vi "Main_Andor_Multi_ver1.vi"() -> ()   [LabVIEW 2014]
doc: "This is the main user interface of the Raman spectroscopy system."
uses:
  C:/Users/light/Desktop/Chuanzhen/Labview/Raman/dll/Thorlabs.MotionControl.Controls.dll
  dll/Thorlabs.MotionControl.Controls.dll
  <userlib>/atmcd64d.llb/AcquisitionMode_mode typedef.ctl
  <userlib>/atmcd64d.llb/ReadMode_mode typedef.ctl
  <userlib>/atmcd64d.llb/Shutter_mode typedef.ctl
  <userlib>/atmcd64d.llb/Shutter_type typedef.ctl
  <userlib>/atmcd64d.llb/TriggerMode_mode typedef.ctl
  TypeDef/GalvoInput.ctl
  <userlib>/atmcd64d.llb/Error Code Enum typedef.ctl
  TypeDef/States.ctl
  TypeDef/StageDeviceOut.ctl
  TypeDef/StageHandleIn.ctl
  <vilib>/Utility/miscctls.llb/LVPoint32TypeDef.ctl
  TypeDef/LaserSpot.ctl
  C:/Users/light/Desktop/Chuanzhen/Labview/Raman/dll/ThorLabs.MotionControl.KCube.DCServoCLI.dll
  dll/ThorLabs.MotionControl.KCube.DCServoCLI.dll
  TypeDef/StageSelect.ctl
  TypeDef/inputImages.ctl
  C:/Users/light/Desktop/Chuanzhen/Labview/Raman/dll/Thorlabs.MotionControl.GenericMotorCLI.dll
  dll/Thorlabs.MotionControl.GenericMotorCLI.dll
panel:
  out "Boolean":bool
  in  "Tab Control":enum32{"Main", "Andor", "Galvo"}(tab)
  in  "Galvo DC":bool
  out "Galvo":bool
  out "Spot Y":dbl
  out "Spot X":dbl
  in  "Box":cluster{"Width":dbl, " Height":dbl}={"Width"=200.0, " Height"=214.0}
  in  "Quit":bool
  out "Height":i32=480
  out "Width":i32=640
  out "FPS":dbl=6.258409738085552
  in  "Blacklevel Offset":i32(slide) min=0 max=255 scale=0.0..255.0
  in  "Frame rate":dbl(slide)=30.0 min=0.5 max=17.288905497022668 step=5.487719298245614e-05 scale=0.5..17.288905497022668 scale format="%^#_3g"
  in  "Pixel clock":i32(slide)=20 min=7 max=86 scale=7.0..86.0
  in  "Exposure time (ms)":dbl(slide)=11.094175438596492 min=0.008982456140350877 max=107.28491228070176 step=0.05487719298245614 scale=0.008982456140350877..107.28491228070176 scale format="%#.3g"
  in  "Edge Filter Enable / Disable":bool
  in  "Edge Filter":i32(ring)=2 items=["High"=1, "Low"=2]
  in  "Blacklevel compensation":bool
  in  "Hotpixel correction 2":bool
  in  "Master Gain":i32(slide) min=0 max=100 scale=0.0..100.0
  in  "Autogain":bool
  out "Bits/Pixel":i32=8
  in  "Camera ID":u32
  in  "Scan Mode":bool
  out "Live video":picture caption="600 x 480"
  in  "Focus":bool
  out "ZoomRatio":dbl format="%#_2g"
  in  "Jog size (um)":dbl=2.0
  out "Delay (s)":dbl=0.9 format="%#_13g"
  out "Focal plane (mm)":dbl
  out "Initialization finished":bool
  in  "Aim":bool
  in  "Pixel Size X (um)":dbl=0.0877
  in  "LaserSpot":bool
  in  "Pixel Size Y (um)":dbl=0.0877
  in  "Snap":bool
  in  "Left":bool
  in  "Right":bool
  in  "Up":bool
  in  "Down":bool
  in  "X axis_R":bool
  in  "X axis_L":bool
  in  "Reset":bool
  out "Z_axis":dbl
  out "X_axis":dbl
  out "Y_axis":dbl
  in  "Y axis_B":bool
  in  "Y axis_F":bool
  in  "Z axis_u":bool
  in  "Z axis_d":bool
  in  "Jogstep of Z axis":T1(radio)=enum."10step"
  in  "MoveTo":bool
  in  "Velocity: X and Y axis":T2(radio)=enum."0.05mm"
  in  "Scan":bool
  in  "Save Path":path=path "C:/Users/light/Desktop/Chuanzhen/test"
  in  "Destination":dbl=12.0
  out "Frame_X":dbl
  out "Frame_Y":dbl
  out "Total_Frame_X":dbl
  out "Total_Frame_Y":dbl
  in  "Galvo Stop":bool
  in  "Galvo Scan":bool
  out "Andor":bool
  in  "Delay/ms":u32=500
  in  "Set":bool
  in  "AndorSnap":bool
  out "SaveStatus":bool
  in  "FilePath":string="C:\\Users\\light\\Desktop\\Chuanzhen\\Image\\ImageReconstruct\\data"
  in  "Exit":bool
  out "ShutDown":cluster{"CoolOff":bool, "ShutDown":bool}
  in  "Mode":T8={"AcqMode"=enum."Single Scan", "ReadMode"=enum."Single-Track", "ShutterMode"=enum."Auto", "GateMode"=enum."TTL High", "TriggerMode"=enum."Internal"}
  in  "AcqSet":T9={"openingtime"=15, "closingtime/ms"=15, "ExposureTime/s"=0.1, "AccumCycTime"=0.0, "AccumCycNum"=1, "KineticNum"=1, "KineticTime"=0.0} {"KineticTime" format="%.5f"; "AccumCycNum" format="%.5f"; "AccumCycTime" format="%.5f"; "ExposureTime/s" format="%.5f"; "closingtime/ms" format="%.2f"; "openingtime" format="%.2f"}
  out "Timing":T10 {"kinetic" format="%.7f"; "accumulate" format="%.7f"; "exposure" format="%.7f"}
  out "SetOut":T11
  in  "MultiTrack":cluster{"StartRow":i32, "EndRow":i32}={"StartRow"=131, "EndRow"=143}
  out "SetStatus":bool
  out "CurrentTemp":i32
  out "DevInit":bool
  out "DevSize":cluster{"xpixels":i32, "ypixels":i32}
  out "HardWVersion":T12
  out "SoftWVersion":T13
  out "Speeds":T14
  in  "TargetTemp":i32=-70
  out "CoolerON":T15
  out "GetStatus":T16
  in  "YOffset":dbl=8.2 caption="Offset"
  in  "XOffset":dbl=4.0 caption="Offset"
  out "Sample Rate":dbl=1000.0 format="%0.2f"
  out "Waveform Graph":waveform(dbl)[](graph)=[{"t0"=timestamp(0 s since 1904-01-01), "dt"=0.001, "Y"=[]}]
  in  "ZOffset":dbl caption="Offset"
  in  "Galvo":T17={"Sample Rate"=50.0, "Sample Clock Source"="OnboardClock", "Max Voltage"=10.0, "Min Voltage"=-10.0, "Physical Channel(s)"="Dev1/ao0,Dev1/ao1,Dev1/ao3"}
  in  "Stage Control":enum32{"X axis", "Y axis", "Z axis"}(tab)
  in  "X axis":refnum<k24>(container)
  in  "Y axis":refnum<k24>(container)
  in  "Z axis":refnum<k24>(container)
  # "Camera Control"
  # "Objective: CFI Plan Fluor ELWD 60x (1.27 NA) \nThe depth of field: 1.78 um\nPixel Size: 0.0877um/px"
  # "Attention: \ndon't click button very fast"
  # "Motor Control"
  # "Aim"
  # "Auto Focus"
  # "Adjust laser spot lightly"
  # "Stage Scan"
  # "Total_Frame"
  # "Current_Frame"
  # "X"
  # "Y"
  # "Focus distance ia about 2mm"
  # "Jogstep:"
  # "0.00003mm/step"
  # "Stepsize:"
  # "Kinetics->SignleTrack"
  # "Galvo Control"
  # "50Hz->1s"
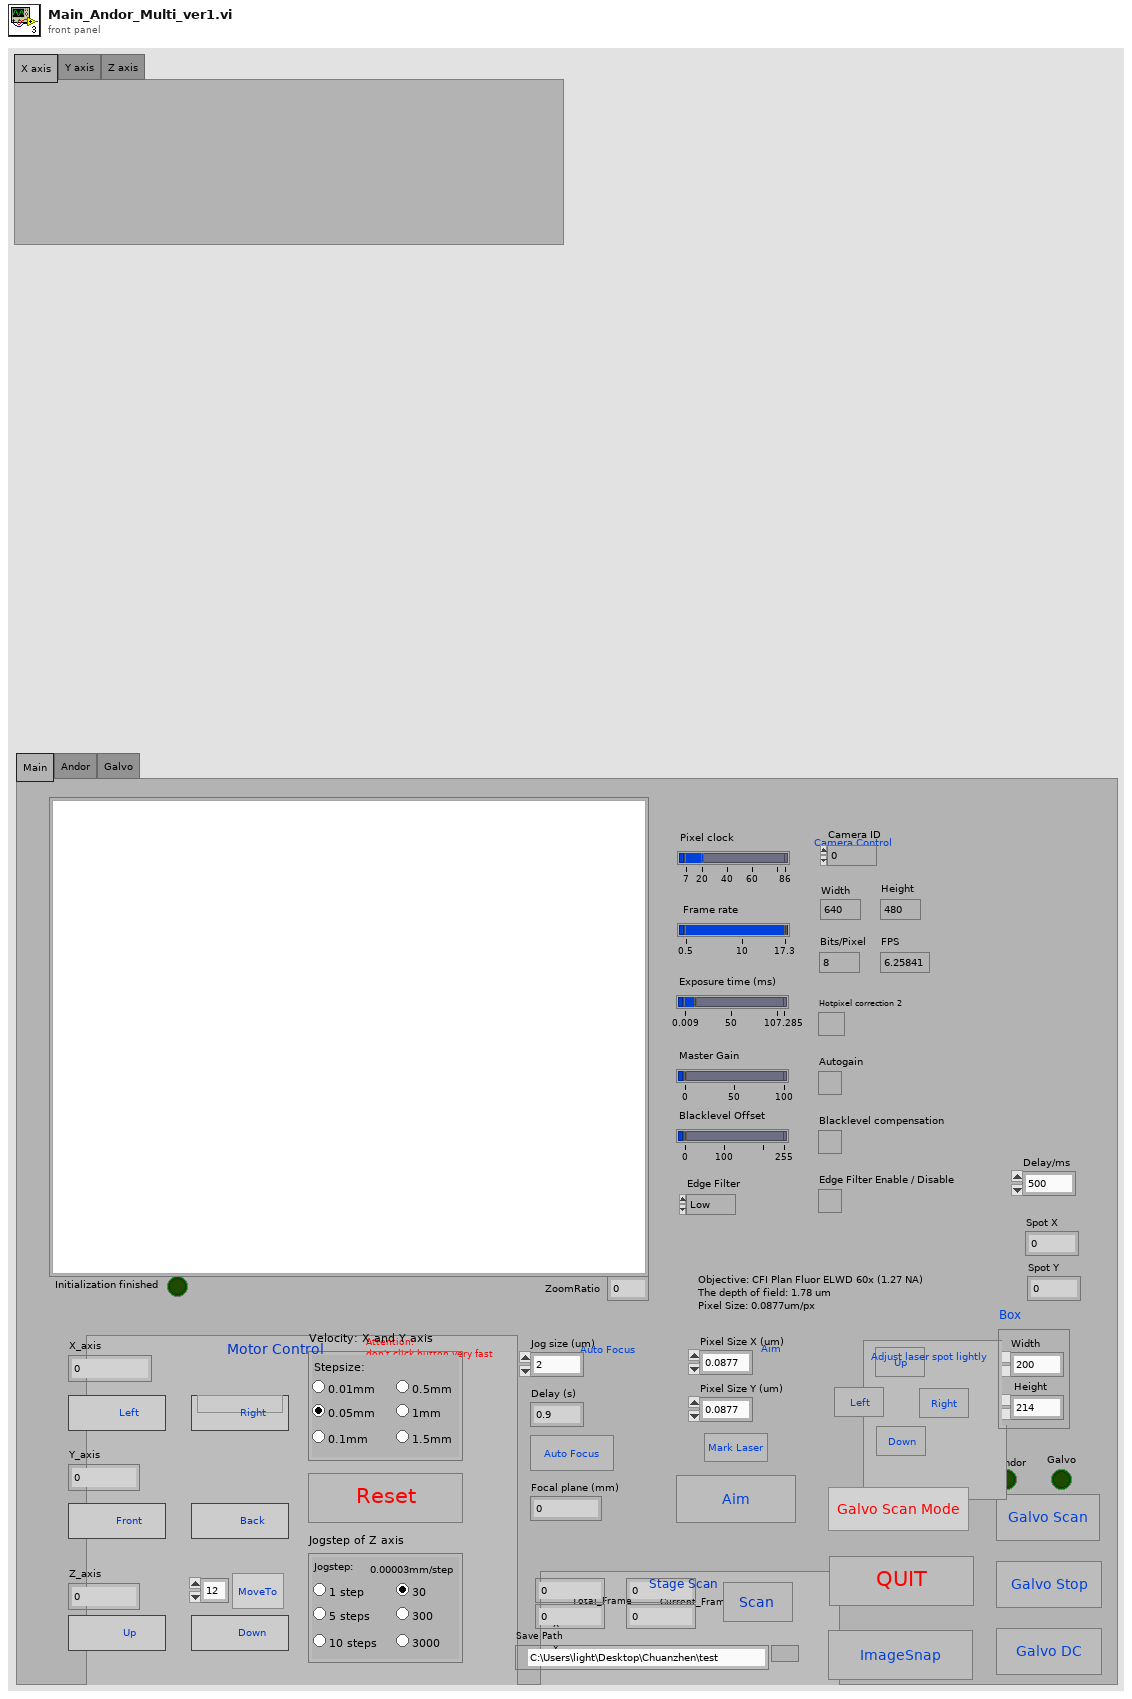
[diagram p1: front panel]
types:
  T1 = enum32{"1step", "2step", "5step", "10step", "15step", "20step"}
  T2 = enum32{"0.01mm", "0.05mm", "0.1mm", "0.5mm", "1mm", "1.5mm"}
  T3 = typedef "AcquisitionMode_mode typedef.ctl" = enum16{"Reserved (0)", "Single Scan", "Accumulate", "Kinetics", "Fast Kinetics", "Run Till Abort", "Reserved (6)", "Reserved (7)", "Reserved (8)", "Time Delayed Integration"}
  T4 = typedef "ReadMode_mode typedef.ctl" = enum16{"Full Vertical Binning", "Multi-Track", "Random-Track", "Single-Track", "Image"}
  T5 = typedef "Shutter_mode typedef.ctl" = enum16{"Auto", "Open", "Close", "N/A (3)", "Open FVB Series", "Open Any Series"}
  T6 = typedef "Shutter_type typedef.ctl" = enum16{"TTL Low", "TTL High"}
  T7 = typedef "TriggerMode_mode typedef.ctl" = enum16{"Internal", "External", "N/A (2)", "N/A (3)", "N/A (4)", "N/A (5)", "External Start", "External Exposure (Bulb)", "N/A (8)", "External FVB EM", "Software", "N/A (11)", "External Charge Shifting"}
  T8 = cluster{"AcqMode":T3, "ReadMode":T4, "ShutterMode":T5, "GateMode":T6, "TriggerMode":T7}
  T9 = cluster{"openingtime":i32, "closingtime/ms":i32, "ExposureTime/s":sgl, "AccumCycTime":sgl, "AccumCycNum":i32, "KineticNum":i32, "KineticTime":sgl}
  T10 = cluster{"exposure":sgl, "accumulate":sgl, "kinetic":sgl}
  T11 = cluster{"Height":i32, "Width":i32, "bottom":i32, "gap":i32}
  T12 = cluster{"PCB":u32, "Flex":u32, "dummy1":u32, "dummy2":u32, "dummy3":u32, "dummy4":u32}
  T13 = cluster{"eprom":u32, "cofFile":u32, "vxdRev":u32, "vxdVer":u32, "dllRev":u32, "dllVer":u32}
  T14 = cluster{"NVS":i32, "VS":i32, "NHS":dbl, "HS":i32}
  T15 = cluster{"SetTemp":bool, "CoolerOn":bool, "Stablized":bool}
  T16 = cluster{"GetDetector":bool, "GetHardVer":bool, "GetNVS":bool, "GetVS":bool, "GetSotfVer":bool, "GetNHS":bool, "GetHS":bool}
  T17 = typedef "GalvoInput.ctl" = cluster{"Sample Rate":dbl, "Sample Clock Source":tag, "Max Voltage":dbl, "Min Voltage":dbl, "Physical Channel(s)":tag}
  T18 = typedef "LaserSpot.ctl" = cluster{"Laser X":dbl, "Laser Y":dbl}
  T19 = cluster{"left":i16, "top":i16, "right":i16, "bottom":i16}
  T20 = typedef "LVPoint32TypeDef.ctl" = cluster{"Horizontal":i32, "Vertical":i32}
  T21 = typedef "StageHandleIn.ctl" = cluster{"Z StageHandle in":refnum<k24>, "X StageHandle in":refnum<k24>, "Y StageHandle in":refnum<k24>}
  T22 = typedef "StageDeviceOut.ctl" = cluster{"Device Z":refnum<k24>, "Device X":refnum<k24>, "Device Y":refnum<k24>}
  T23 = typedef "States.ctl" = enum16{"Initialize", "CMOS live", "Shut down"}
  T24 = enum8{"Enabled", "Disabled", "Disabled and Grayed Out"}
  T25 = cluster{"Width":u16, "Style":enum32{"Solid", "Dash", "Dot", "DashDot", "DashDotDot"}}
  T26 = typedef "StageSelect.ctl" = enum16{"X axis", "Y axis", "Z axis"}
  T27 = typedef "inputImages.ctl" = cluster{"Image2":u8[][], "Image3":u8[][], "Image4":u8[][], "Image1":u8[][]}
  T28 = typedef "StageHandleOut.ctl" = cluster{"Z StageHandle out":refnum<k24>, "X StageHandle out":refnum<k24>, "Y StageHandle out":refnum<k24>}
  T29 = typedef "LVBoundsTypeDef.ctl" = cluster{"Width":u32, "Height":u32}
  T30 = typedef "imagedata.ctl" = cluster{"image type":i32, "image depth":i32, "image":u8[], "mask":u8[], "colors":u32[], "Rectangle":cluster{"left":i16, "top":i16, "right":i16, "bottom":i16}}
  T31 = typedef "LVPositionTypeDef.ctl" = cluster{"Left":i32, "Top":i32}
  T32 = typedef "Error Code Enum typedef.ctl" = enum32{"N/A (0)", "DRV_ERROR_CODES", "DRV_SUCCESS", "DRV_VXDNOTINSTALLED", "DRV_ERROR_SCAN", "DRV_ERROR_CHECK_SUM", "DRV_ERROR_FILELOAD", "DRV_UNKNOWN_FUNC", "DRV_ERROR_VXD_INIT", "DRV_ERROR_ADDRESS", "DRV_ERROR_PAGELOCK", "DRV_ERROR_PAGEUNLOCK", "DRV_ERROR_BOARDTEST", "DRV_ERROR_ACK", "DRV_ERROR_UP_FIFO", "DRV_ERROR_PATTERN", "N/A (16)", "DRV_ACQUISITION_ERRORS", "DRV_ACQ_BUFFER", "DRV_ACQ_DOWNFIFO_FULL", "DRV_PROC_UNKONWN_INSTRUCTION", "DRV_ILLEGAL_OP_CODE", "DRV_KINETIC_TIME_NOT_MET", "DRV_ACCUM_TIME_NOT_MET", "DRV_NO_NEW_DATA", "N/A (25)", "DRV_SPOOLERROR", "N/A (27)", "N/A (28)", "N/A (29)", "N/A (30)", "N/A (31)", "N/A (32)", "DRV_TEMPERATURE_CODES", "DRV_TEMPERATURE_OFF", "DRV_TEMPERATURE_NOT_STABILIZED", "DRV_TEMPERATURE_STABILIZED", "DRV_TEMPERATURE_NOT_REACHED", "DRV_TEMPERATURE_OUT_RANGE", "DRV_TEMPERATURE_NOT_SUPPORTED", "DRV_TEMPERATURE_DRIFT", "N/A (41)", "N/A (42)", "N/A (43)", "N/A (44)", "N/A (45)", "N/A (46)", "N/A (47)", "N/A (48)", "DRV_GENERAL_ERRORS", "DRV_INVALID_AUX", "DRV_COF_NOTLOADED", "DRV_FPGAPROG", "DRV_FLEXERROR", "DRV_GPIBERROR", "N/A (55)", "N/A (56)", "N/A (57)", "N/A (58)", "N/A (59)", "N/A (60)", "N/A (61)", "N/A (62)", "N/A (63)", "DRV_DATATYPE", "DRV_DRIVER_ERRORS", "DRV_P1INVALID", "DRV_P2INVALID", "DRV_P3INVALID", "DRV_P4INVALID", "DRV_INIERROR", "DRV_COFERROR", "DRV_ACQUIRING", "DRV_IDLE", "DRV_TEMPCYCLE", "DRV_NOT_INITIALIZED", "DRV_P5INVALID", "DRV_P6INVALID", "DRV_INVALID_MODE", "DRV_INVALID_FILTER", "DRV_I2CERRORS", "DRV_I2CDEVNOTFOUND", "DRV_I2CTIMEOUT", "DRV_P7INVALID", "N/A (84)", "N/A (85)", "N/A (86)", "N/A (87)", "N/A (88)", "N/A (89)", "DRV_IOCERROR", "DRV_VRMVERSIONERROR"}
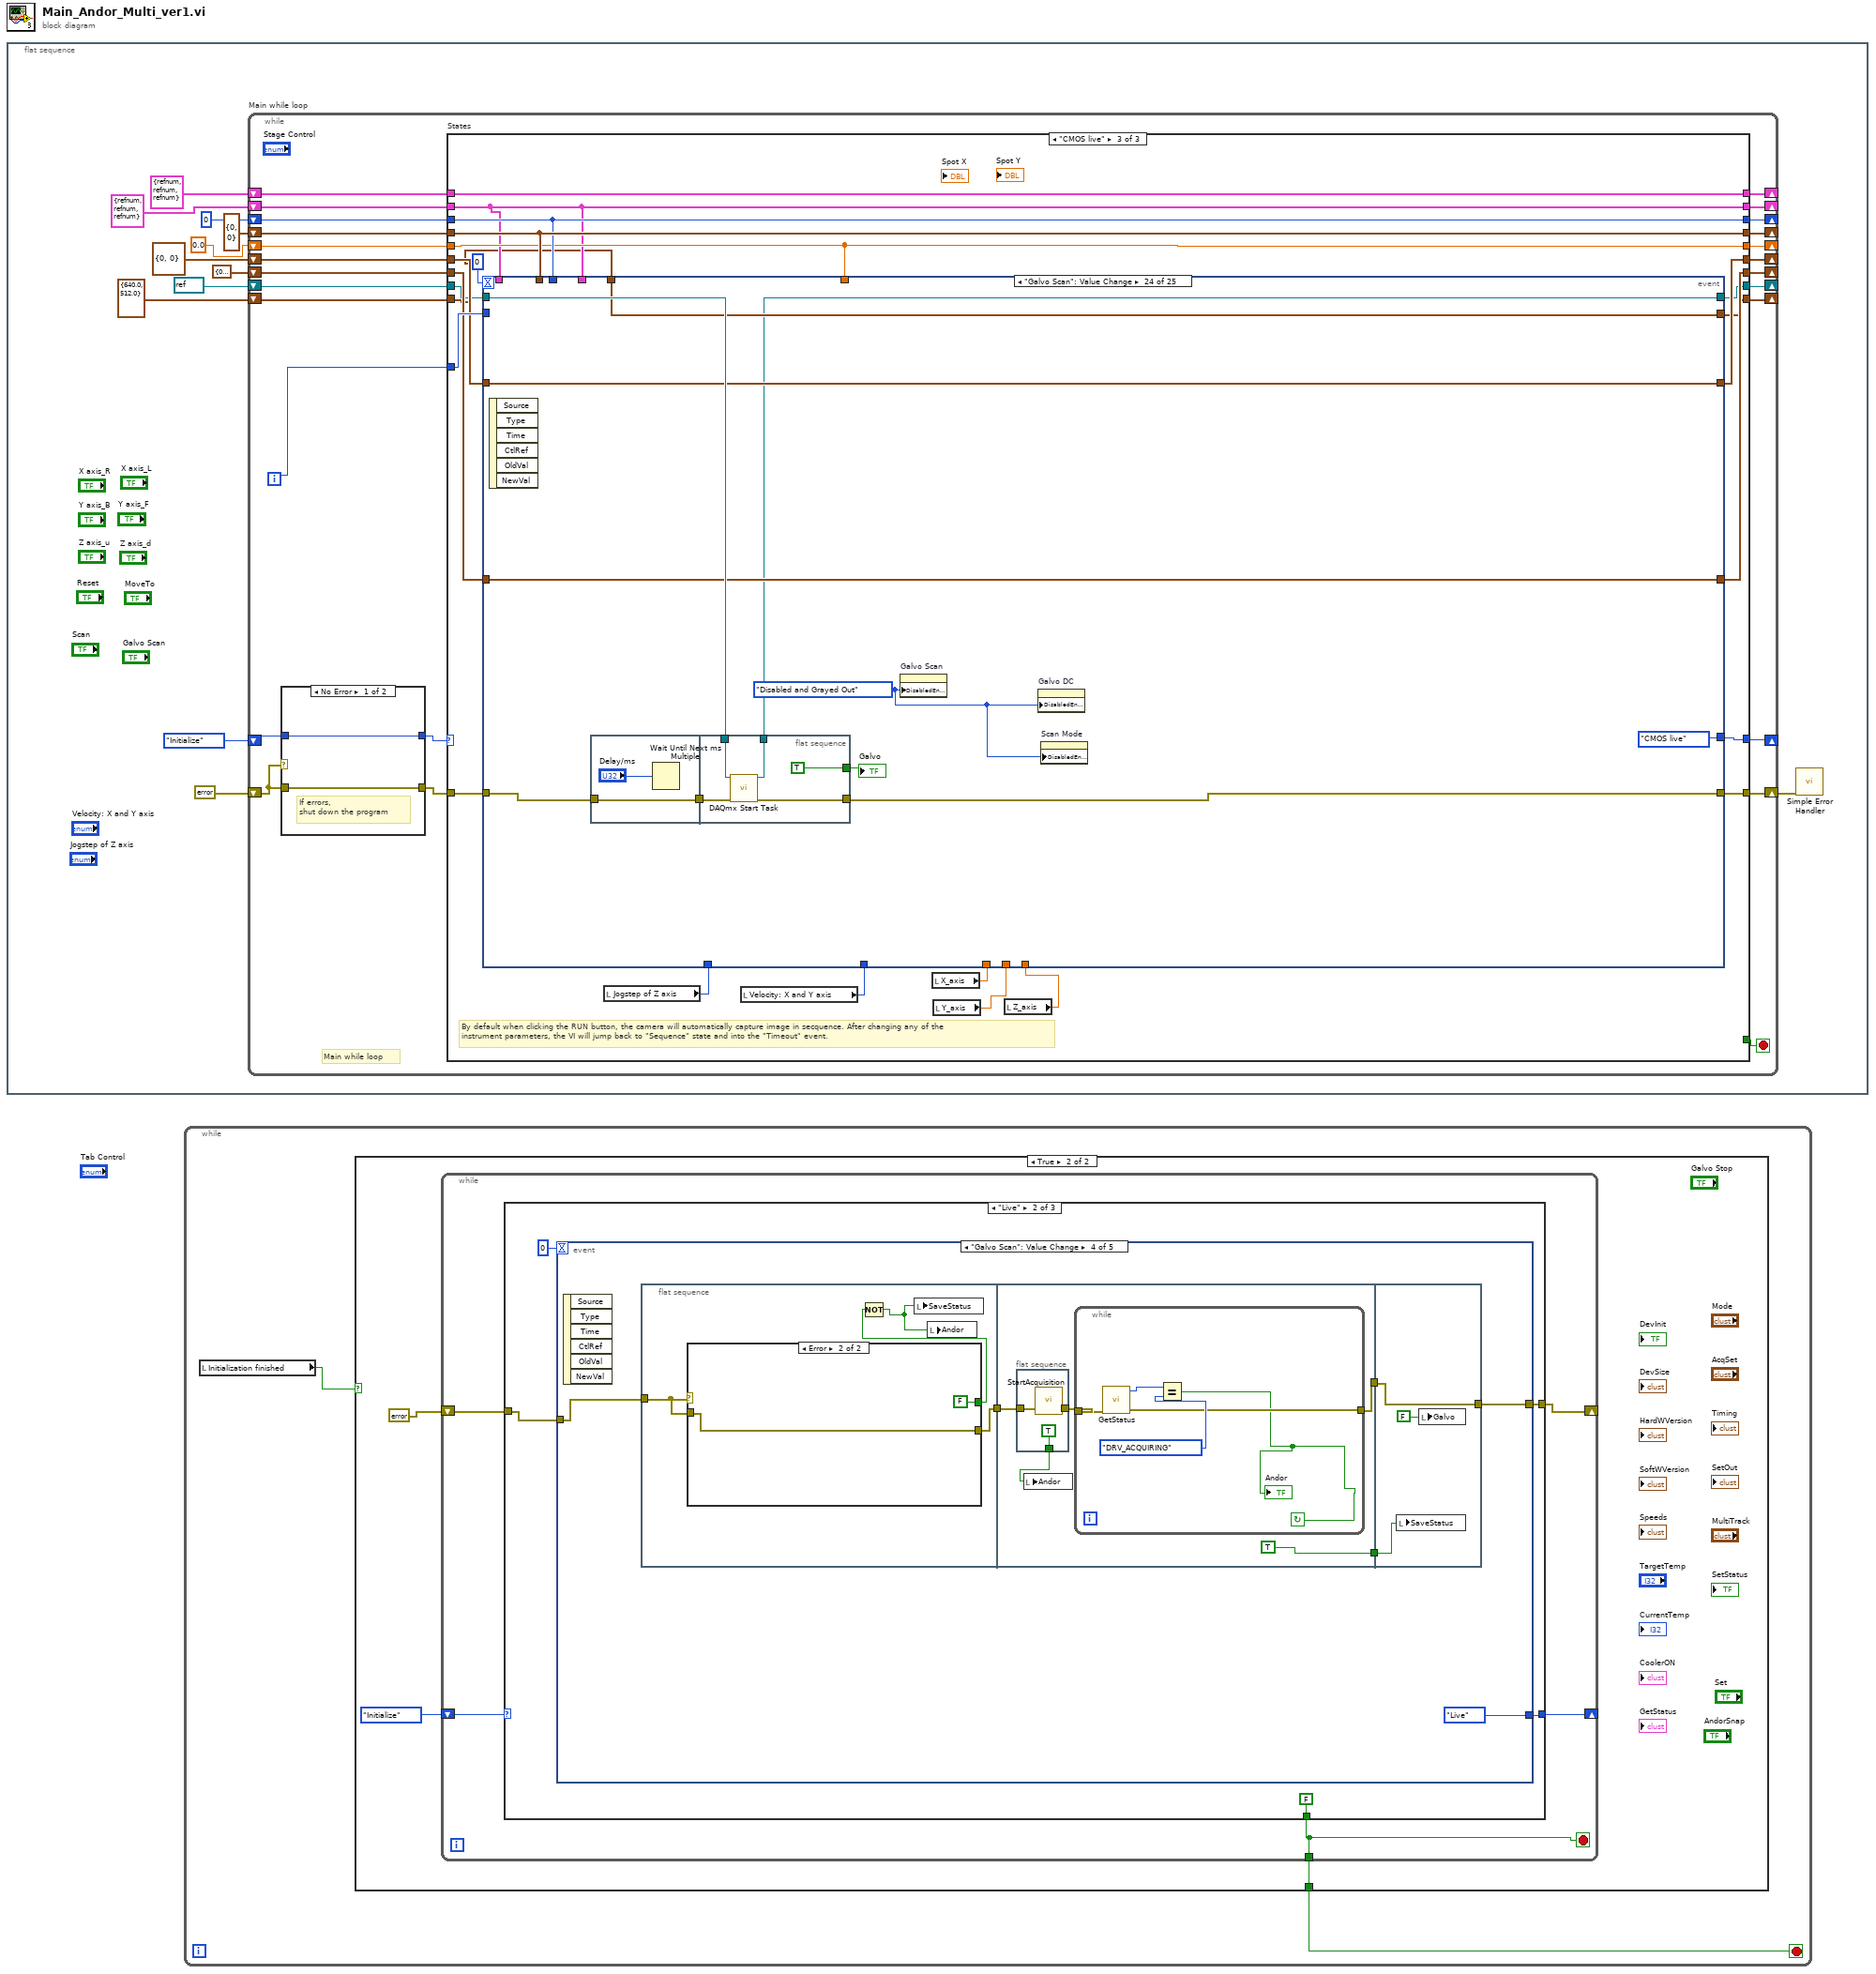
[diagram p0: block diagram]
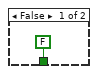
[diagram p2: hidden frame]
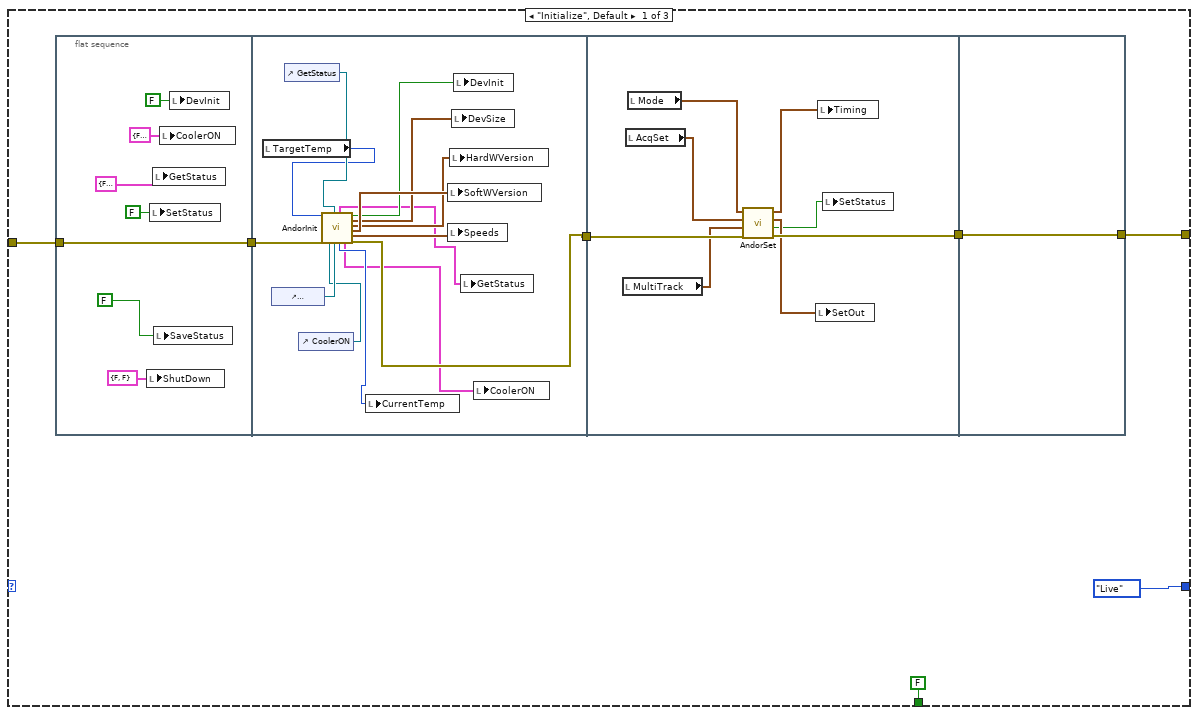
[diagram p3: hidden frame]
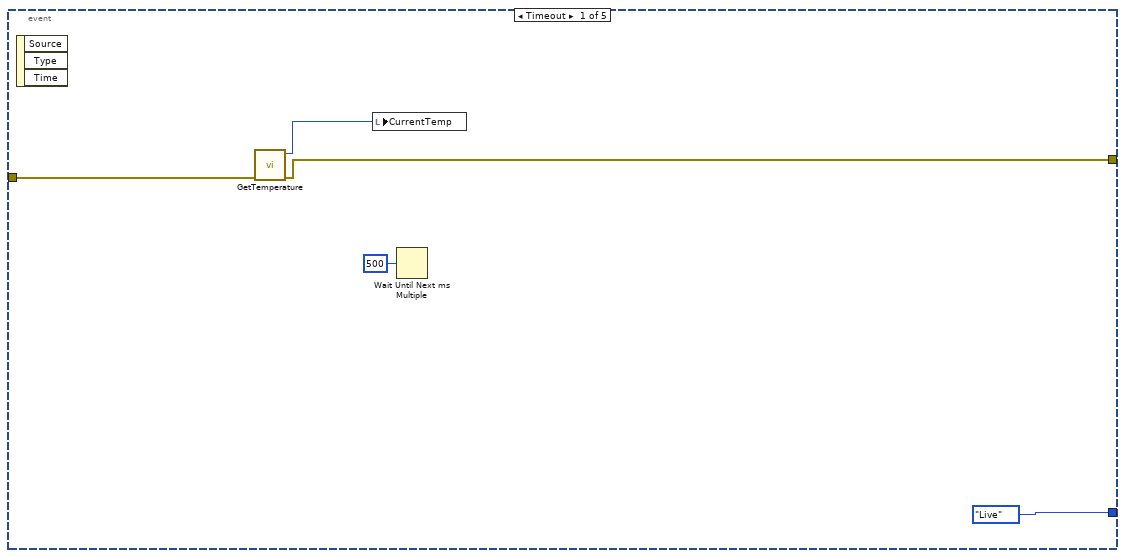
[diagram p4: hidden frame]
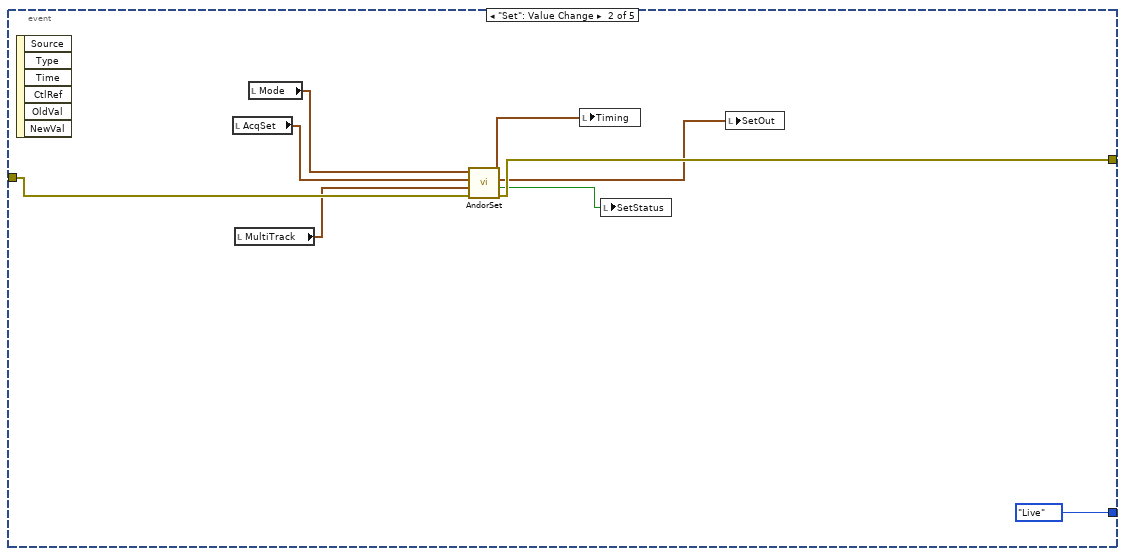
[diagram p5: hidden frame]
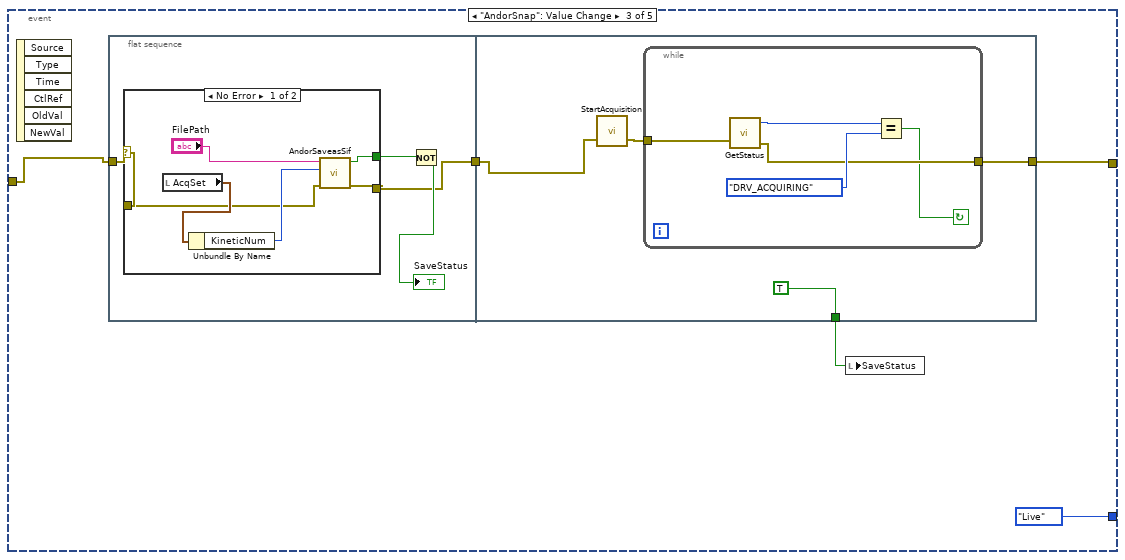
[diagram p6: hidden frame]
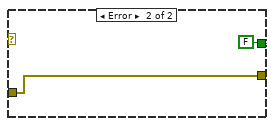
[diagram p7: hidden frame]
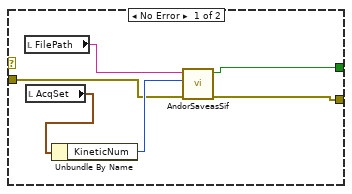
[diagram p8: hidden frame]
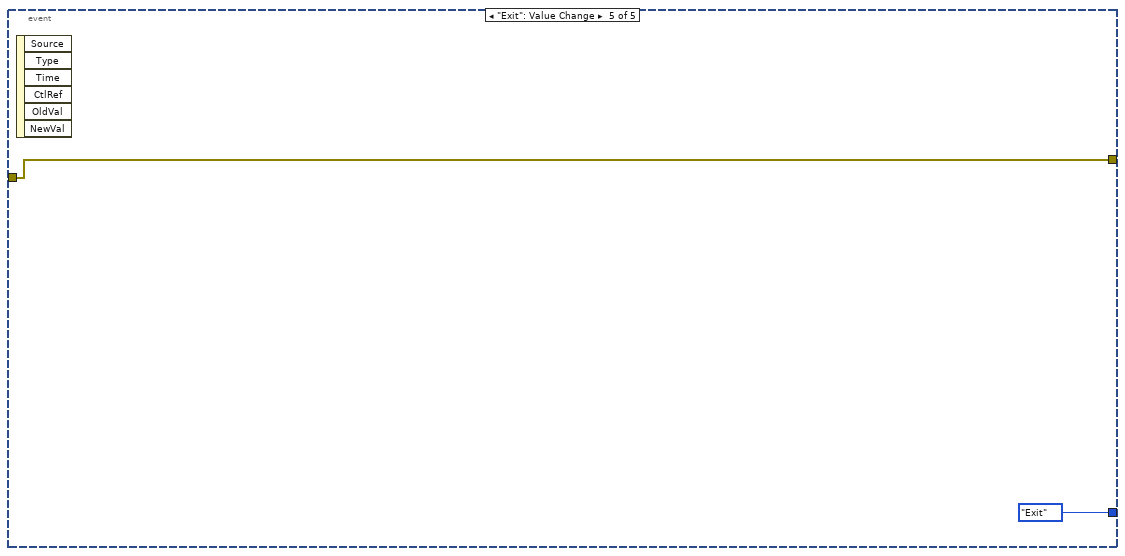
[diagram p9: hidden frame]
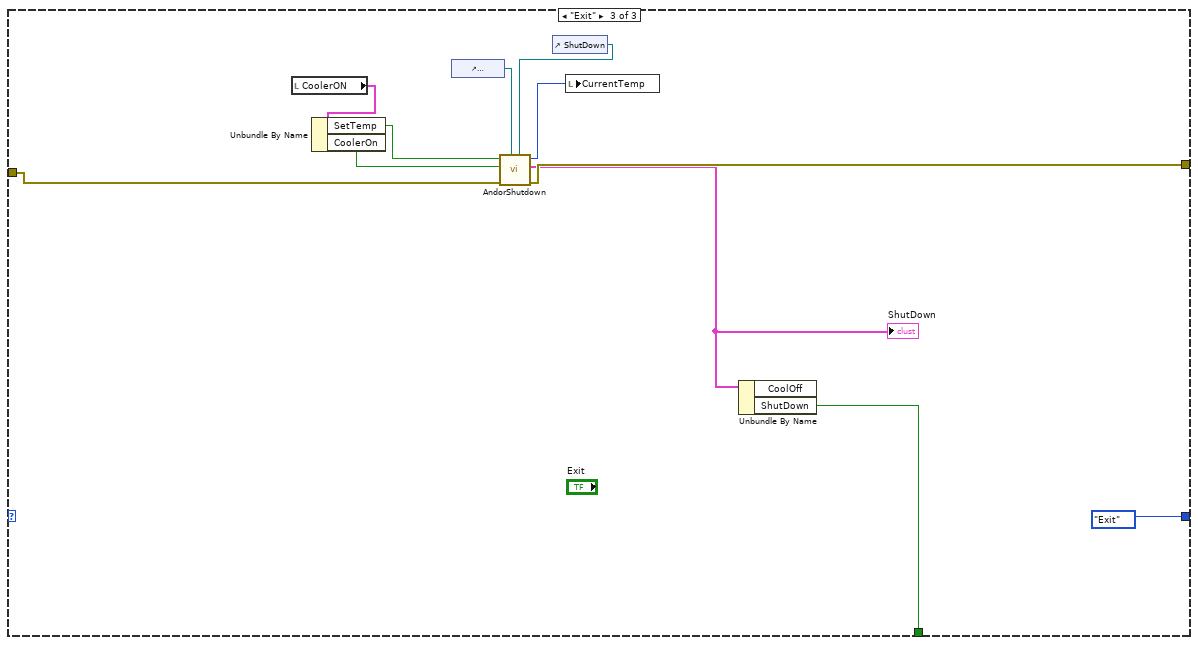
[diagram p10: hidden frame]
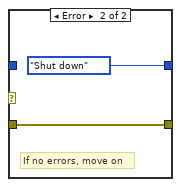
[diagram p11: hidden frame]
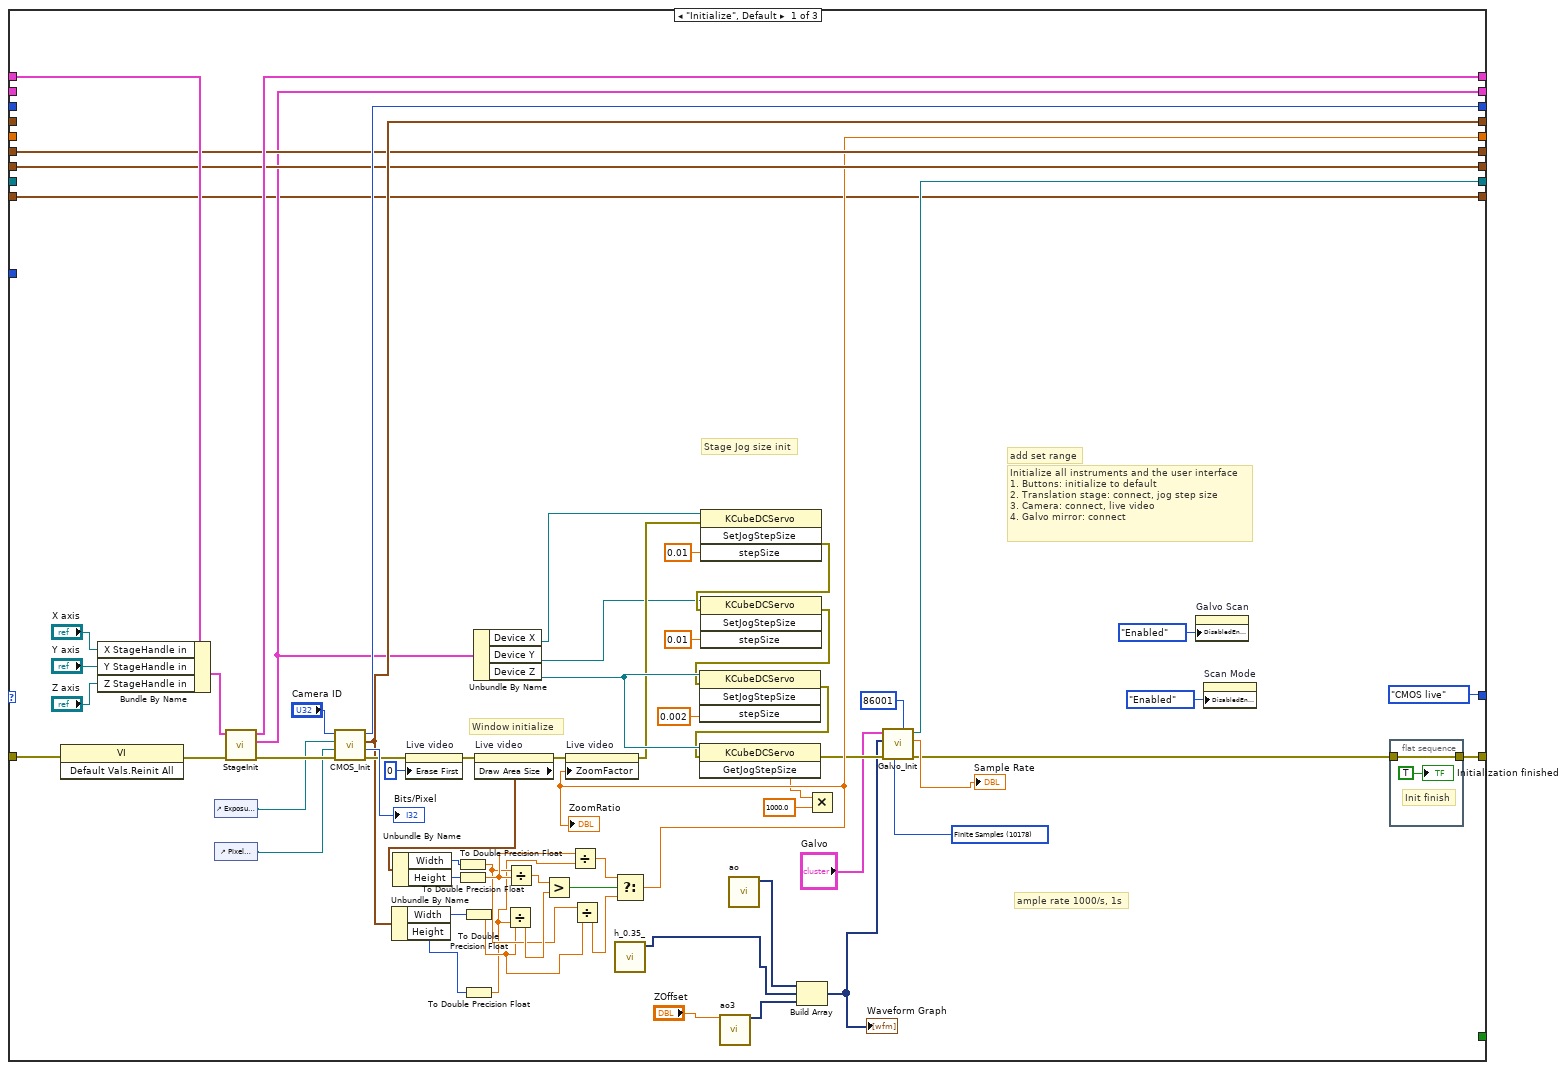
[diagram p12: hidden frame]
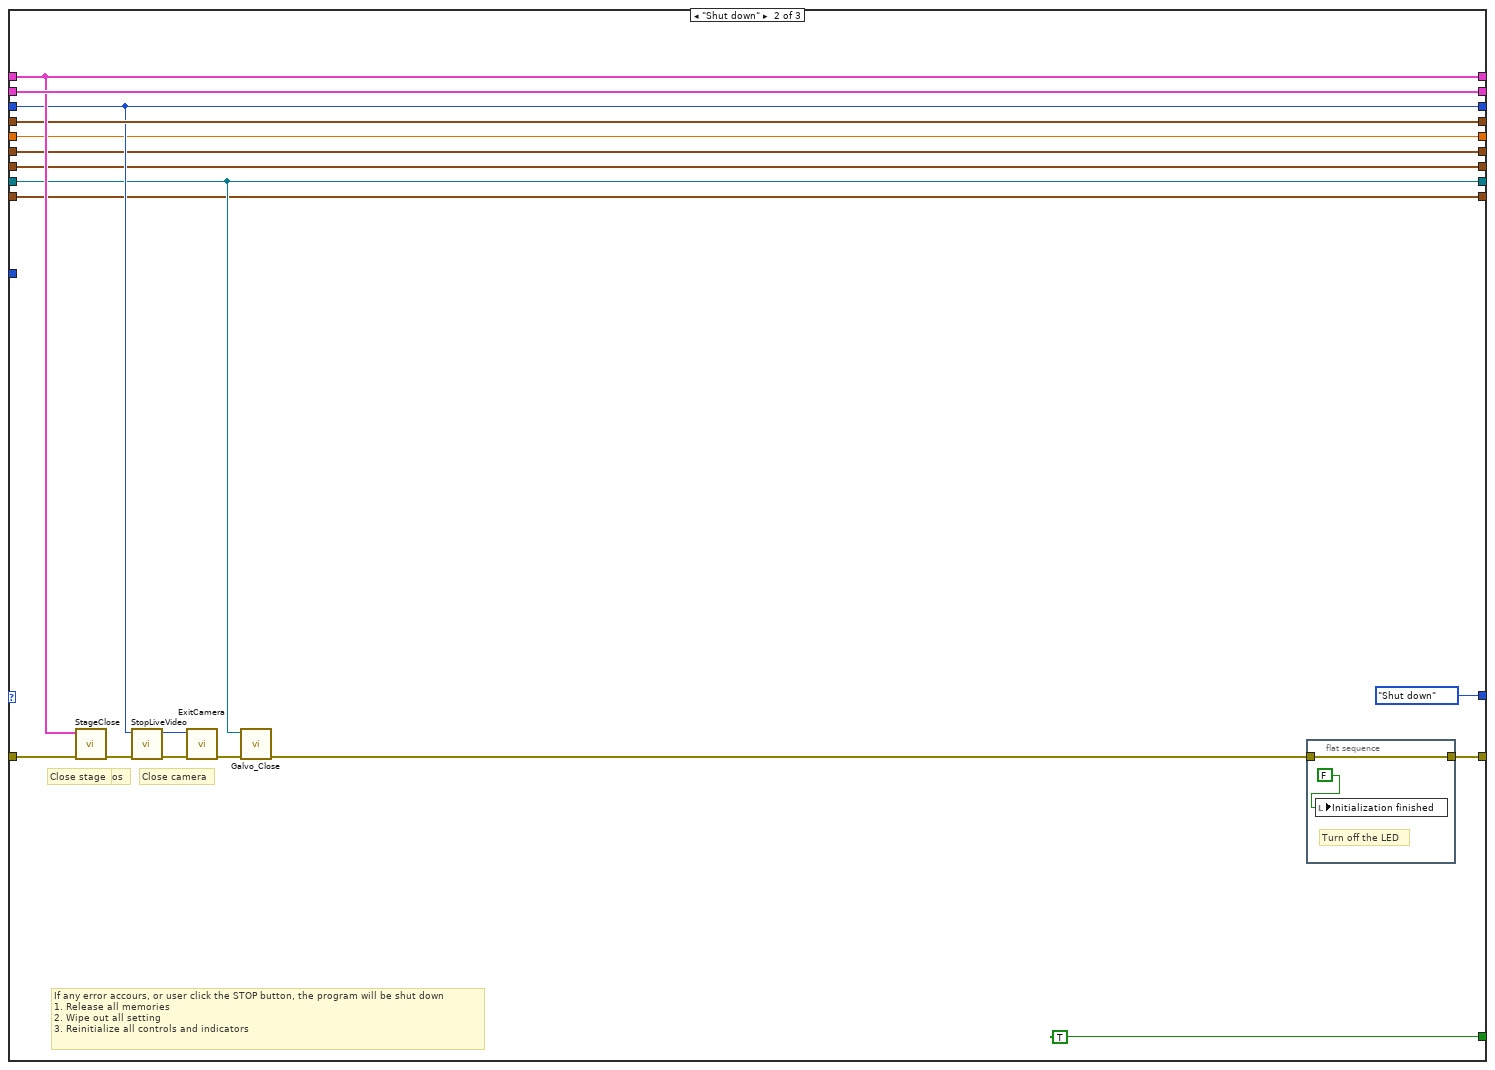
[diagram p13: hidden frame]
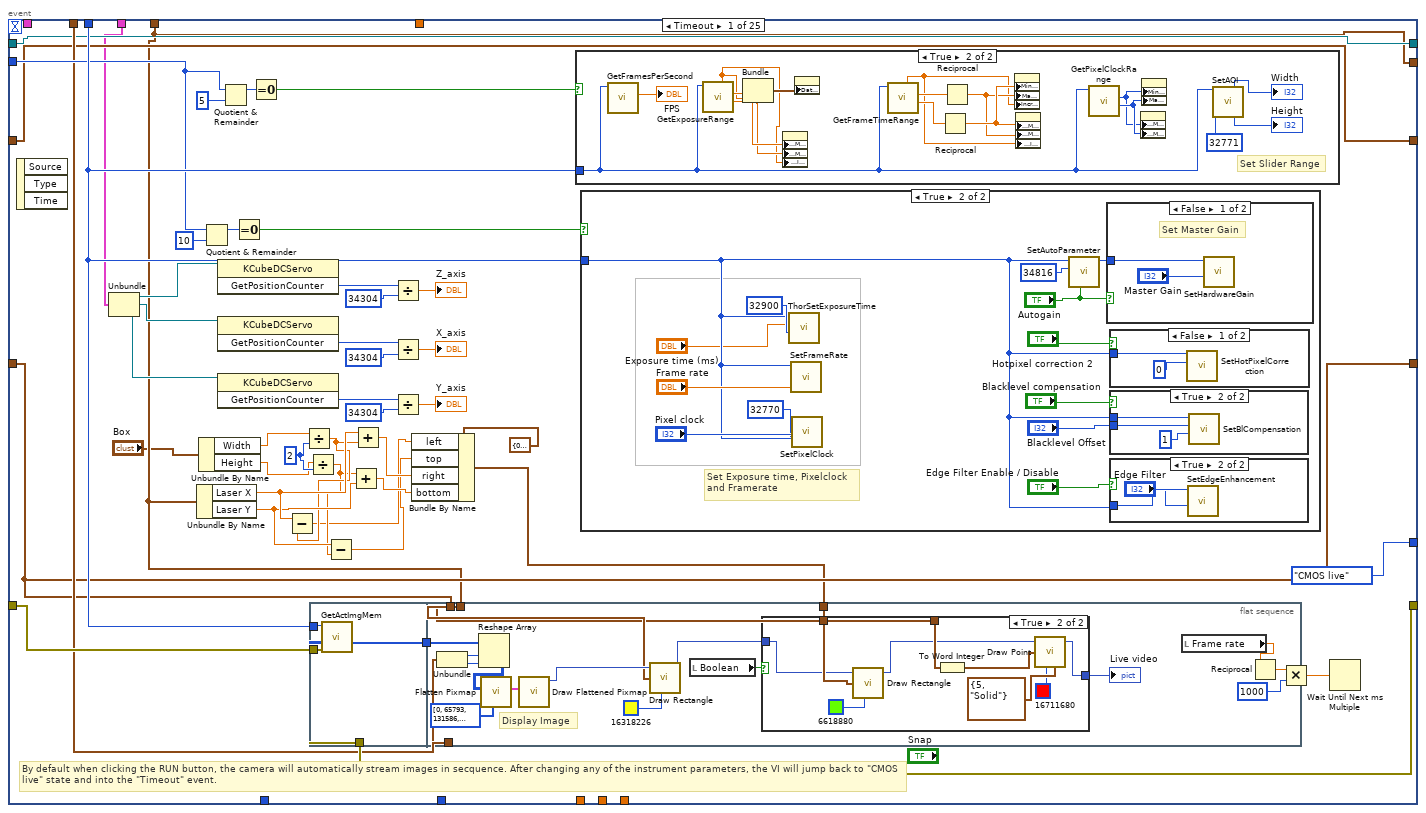
[diagram p14: hidden frame]
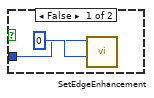
[diagram p16: hidden frame]
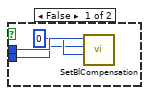
[diagram p17: hidden frame]
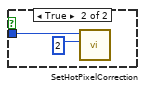
[diagram p18: hidden frame]
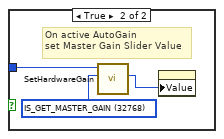
[diagram p19: hidden frame]
diagram:
  n1 = flat-sequence {
    frame #0 {
      n2 = while "Main while loop" {
        shift-right: [w33] -> _
        shift-left: States."Initialize" -> [w38]
        shift-right: [w36] -> w10
        shift-left: errorcluster {"status"=FALSE, "code"=0, "source"=""} ("error out") -> [w32]
        shift-right: [w30] -> _
        shift-left: T21 {"Z StageHandle in"=refnum, "X StageHandle in"=refnum, "Y StageHandle in"=refnum} ("StageHandle In") -> [w31]
        shift-right: [w29] -> _
        shift-left: T22 {"Device Z"=refnum, "Device X"=refnum, "Device Y"=refnum} ("Device Out") -> [w28]
        shift-right: [w27] -> _
        shift-left: u32 0 ("CMOS Handle Out") -> [w26]
        shift-right: [w24] -> _
        shift-left: cluster{"Height":i32, "Width":i32} {"Height"=0, "Width"=0} ("WidthAndHeight") -> [w23]
        shift-right: [w22] -> _
        shift-left: 0.0 -> [w17]
        shift-right: [w21] -> _
        shift-left: T20 {"Horizontal"=0, "Vertical"=0} ("Coords") -> [w20]
        shift-right: [w19] -> _
        shift-left: T19 {"left"=0, "top"=0, "right"=0, "bottom"=0} ("rect") -> [w18]
        shift-right: [w16] -> _
        shift-left: refnum<k21> refnum ("task out") -> [w15]
        shift-right: [w14] -> _
        shift-left: T18 {"Laser X"=640.0, "Laser Y"=512.0} ("LaserSpot 2") -> [w13]
        i -> [w25]
        stop <- w34 stop-if-true
        # "Main while loop"
        n3 = case shown="No Error" w32 {
          tunnel: w32 -> [w40 w42]
          tunnel: [w40 w42] -> w35
          tunnel: w38 -> [w39 _]
          tunnel: [w39 States."Shut down"] -> w37
          frame No Error {
            # "If errors,\nshut down the program"
          }
          frame Error {
            # "If no errors, move on"
          }
        }
        n4 = case "States" shown="\"CMOS live\"" w37 {
          tunnel: [w66 w115 w150] -> w36
          tunnel: w35 -> [w107 w125 w151]
          tunnel: [_ TRUE _] -> w34
          tunnel: [States."CMOS live" States."Shut down" w152] -> w33
          tunnel: w31 -> [w105 w124 w153]
          tunnel: [w104 w124 w153] -> w30
          tunnel: [w71 w126 w140] -> w29
          tunnel: w28 -> [_ w126 w140]
          tunnel: [w98 w119 w146] -> w27
          tunnel: w26 -> [_ w119 w146]
          tunnel: w25 -> [_ _ w148]
          tunnel: [w79 w123 w147] -> w24
          tunnel: w23 -> [_ w123 w147]
          tunnel: [w72 w118 w141] -> w22
          tunnel: w17 -> [_ w118 w141]
          tunnel: [w74 w117 w145] -> w21
          tunnel: w20 -> [w74 w117 w144]
          tunnel: [w73 w116 w143] -> w19
          tunnel: w18 -> [w73 w116 w142]
          tunnel: [w54 w113 w138] -> w16
          tunnel: w15 -> [_ w113 w139]
          tunnel: [w50 w111 w137] -> w14
          tunnel: w13 -> [w50 w111 w136]
          frame "Initialize", Default {
            w46 = 10178 items=["Finite Samples"=10178, "Continuous Samples"=10123, "Hardware Timed Single Point"=12522] ("Sample Mode")
            # "ample rate 1000/s, 1s"
            # "add set range"
            # "Stage Jog size init"
            # "Window initialize"
            # "Initialize all instruments and the user interface\n1. Buttons: initialize to default\n2. Translation stage: connect, jog step size\n3. Camera: connect, live video\n4. Galvo mirror: connect"
            n5 = invoke class="VI" method="Default Vals.Reinit All"(error in=w107) -> (error out=w106:errorcluster)  [unwired: 2 in, 2 out]
            n6 = Bundle By Name(cluster=w105, "X StageHandle in"="X axis", "Y StageHandle in"="Y axis", "Z StageHandle in"="Z axis") -> (w103:T21)
            n7 = control-ref of="Exposure time (ms)"() -> (w97:refnum<vi>)
            n8 = control-ref of="Pixel clock"() -> (w96:refnum<vi>)
            n9 = call "StageInit.vi"("error in (no error)"=w106, "StageHandle In"=w103) -> ("error out"=w99:errorcluster, "Device Out"=w71:T22, "StageHandle Out"=w104:T28)  [unwired: 7 in]
            n10 = call "CMOS_Init.vi"("error in"=w99, "Pixel clock"=w96, "Exposure time"=w97, "Camera ID"="Camera ID") -> ("error out"=w93:errorcluster, "Bits/Pixel"=→"Bits/Pixel":i32, "WidthAndHeight"=w79:cluster{"Height":i32, "Width":i32}, "CMOS Handle Out"=w98:u32)  [unwired: 3 in]
            n11 = Unbundle By Name(w79) -> ("Width"=w78:i32, "Height"=w77:i32)
            n12 = property on="Live video" class="Pict"(error in=w93, "Erase First"=u8 0) -> (error out=w81:errorcluster)  [unwired: 1 in, 1 out]
            n13 = To Double Precision Float(number=w78) -> (double precision float=w76:dbl)
            n14 = To Double Precision Float(number=w77) -> (double precision float=w75:dbl)
            n15 = Unbundle By Name(w71) -> ("Device X"=w59:refnum<k24>, "Device Y"=w58:refnum<k24>, "Device Z"=w69:refnum<k24>)
            n16 = property on="Live video" class="Pict"(error in=w81) -> (error out=w80:errorcluster, "Draw Area Size"=w91:T29)  [unwired: 1 in, 1 out]
            n17 = Unbundle By Name(w91) -> ("Width"=w89:u32, "Height"=w90:u32)
            n18 = To Double Precision Float(number=w89) -> (double precision float=w83:dbl)
            n19 = To Double Precision Float(number=w90) -> (double precision float=w85:dbl)
            n20 = Divide(x=w76, y=w75) -> (x/y=w86:dbl)
            n21 = Divide(x=w83, y=w85) -> (x/y=w88:dbl)
            n22 = Greater?(x=w88, y=w86) -> (0:w87:bool)
            n23 = Divide(x=w85, y=w75) -> (x/y=w84:dbl)
            n24 = Divide(x=w83, y=w76) -> (x/y=w82:dbl)
            n25 = Select(t=w84, s=w87, f=w82) -> (s? t:f=w72:dbl)
            "ZoomRatio" <- w72
            n26 = property on="Live video" class="Pict"(error in=w80, "ZoomFactor"=w72) -> (error out=w62:errorcluster)  [unwired: 1 in, 1 out]
            n27 = call "h_0.35_"() -> ("Signal"=w44:dynamicdata)  [unwired: 9 in, 2 out]
            n28 = invoke class="KCubeDCServo" method="SetJogStepSize"(reference=w59, error in=w62, "stepSize"=0.01) -> (error out=w61:errorcluster)  [unwired: 1 in, 3 out]
            n29 = invoke class="KCubeDCServo" method="SetJogStepSize"(reference=w58, error in=w61, "stepSize"=0.01) -> (error out=w60:errorcluster)  [unwired: 1 in, 3 out]
            n30 = invoke class="KCubeDCServo" method="SetJogStepSize"(reference=w69, error in=w60, "stepSize"=0.002) -> (error out=w68:errorcluster)  [unwired: 1 in, 3 out]
            n31 = invoke class="KCubeDCServo" method="GetJogStepSize"(reference=w69, error in=w68) -> (error out=w57:errorcluster, "GetJogStepSize"=w67:dbl)  [unwired: 1 in, 1 out]
            n32 = call "ao3"("Offset"="ZOffset") -> ("DC"=w52:dynamicdata)  [unwired: 13 in, 1 out]
            n33 = call "ao"() -> ("Signal"=w49:dynamicdata)  [unwired: 9 in, 2 out]
            n34 = Build Array(w49, w44, w52) -> (w51:dynamicdata[])
            "Waveform Graph" <- w51
            n35 = Multiply(x=w67, y=1000.0) -> ()  [unwired: 1 out]
            n36 = call "Galvo_Init.vi"("Sample Mode"=w46, "samples per channel"=86001, "error in"=w57, "Signal array"=w51, "Galvo_Input"="Galvo") -> ("error out"=w53:errorcluster, "Actual Sample Rate"=→"Sample Rate":dbl, "task out"=w54:refnum<k21>)  [unwired: 4 in]
            n37 = property on="Galvo Scan" class="Bool"("DisabledEnum"=T24."Enabled" ("Disabled")) -> ()  [unwired: 2 in, 2 out]
            n38 = property on="Scan Mode" class="Bool"("DisabledEnum"=T24."Enabled" ("Disabled")) -> ()  [unwired: 2 in, 2 out]
            n39 = flat-sequence {
              tunnel: w53 -> [w110]
              tunnel: [w110] -> w66
              frame #0 {
                # "Init finish"
                "Initialization finished" <- TRUE ("Initialization finished")
              }
            }
          }
          frame "Shut down" {
            # "Close 3 galvos"
            # "Close camera"
            # "Close stage"
            # "If any error accours, or user click the STOP button, the program will be shut down\n1. Release all memories\n2. Wipe out all setting\n3. Reinitialize all controls and indicators"
            n40 = call "StageClose.vi"("error in (no error)"=w125, "StageHandle In"=w124) -> ("error out"=w122:errorcluster)  [unwired: 9 in]
            n41 = call "StopLiveVideo.vi"("error in"=w122, "Camera Handle In"=w119) -> ("error out"=w121:errorcluster, "Camera Handle Out"=w120:u32)  [unwired: 8 in]
            n42 = call "ExitCamera.vi"("error in"=w121, "Camera Handle In"=w120) -> ("error out"=w114:errorcluster)  [unwired: 9 in]
            n43 = call "Galvo_Close.vi"("error in"=w114, "task/channels in"=w113) -> ("error out"=w112:errorcluster)  [unwired: 9 in]
            n44 = flat-sequence {
              tunnel: w112 -> [w130]
              tunnel: [w130] -> w115
              frame #0 {
                # "Turn off the LED"
                n45 = local write "Initialization finished"(FALSE ("Initialization finished")) -> ()
              }
            }
          }
          frame "CMOS live" {
            # "By default when clicking the RUN button, the camera will automatically capture image in secquence. After changing any of the \ninstrument parameters, the VI will jump back to \"Sequence\" state and into the \"Timeout\" event."
            n46 = local read "Jogstep of Z axis"() -> (w131:T1)
            n47 = local read "Velocity: X and Y axis"() -> (w135:T2)
            n48 = local read "X_axis"() -> (w134:dbl)
            n49 = local read "Y_axis"() -> (w133:dbl)
            n50 = local read "Z_axis"() -> (w132:dbl)
            n51 = event shown="[23] \"Galvo Scan\": Value Change" {
              selector: _ -> [_ _ _ _ _ _ _ _ _ _ _ _ _ _ _ _ _ _ _ _ _ _ _ _ _]
              dyn-events: _ -> [_ _ _ _ _ _ _ _ _ _ _ _ _ _ _ _ _ _ _ _ _ _ _ _ _]
              timeout: 0 -> [_ _ _ _ _ _ _ _ _ _ _ _ _ _ _ _ _ _ _ _ _ _ _ _ _]
              tunnel: [States."CMOS live" States."CMOS live" States."CMOS live" States."CMOS live" States."CMOS live" States."CMOS live" States."CMOS live" States."CMOS live" States."CMOS live" States."CMOS live" States."CMOS live" States."CMOS live" States."CMOS live" States."CMOS live" States."CMOS live" States."Shut down" States."CMOS live" States."CMOS live" States."CMOS live" States."CMOS live" States."CMOS live" States."CMOS live" States."CMOS live" States."CMOS live" States."CMOS live"] -> w152
              tunnel: w151 -> [w190 w288 w330 w599 w622 w647 w670 w695 w719 w739 w740 w755 w776 w792 w800 w832 w879 w949 w971 w982 w993 w1004 w1015 w1024 w1035]
              tunnel: [w189 w288 w329 w599 w622 w647 w670 w695 w719 w739 w740 w759 w770 w792 w800 w832 w851 w950 w971 w982 w993 w1004 w1015 w1019 w1036] -> w150
              tunnel: w146 -> [w188 _ w328 _ _ _ _ _ _ _ w749 _ _ _ _ _ w876 _ _ _ _ _ _ _ _]
              tunnel: w148 -> [w187 _ _ _ _ _ _ _ _ _ _ _ _ _ _ _ _ _ _ _ _ _ _ _ _]
              tunnel: w147 -> [w186 _ w327 _ _ _ _ _ _ _ w742 _ _ _ _ _ w875 _ _ _ _ _ _ _ _]
              tunnel: [w184 w287 w339 w598 w621 w646 w669 w694 w718 w738 w753 w768 w788 w794 w802 w831 w881 w953 w970 w981 w992 w1003 w1014 w1022 w1041] -> w145
              tunnel: w144 -> [w184 w287 w339 w598 w621 w646 w669 w694 w718 w738 w753 w768 w788 _ w802 w831 w881 w953 w970 w981 w992 w1003 w1014 w1022 w1041]
              tunnel: [w185 w286 w325 w597 w620 w645 w668 w693 w717 w737 w752 w767 w787 w793 w805 w830 w874 w948 w959 w980 w991 w1002 w1013 w1021 w1040] -> w143
              tunnel: w142 -> [w185 w286 w325 w597 w620 w645 w668 w693 w717 w737 w752 w767 w787 w793 _ w830 w874 w948 w959 w980 w991 w1002 w1013 w1021 w1040]
              tunnel: w141 -> [_ _ _ _ _ _ _ _ _ _ _ _ _ _ w804 _ _ _ _ _ _ _ _ _ _]
              tunnel: w140 -> [_ _ _ _ _ _ _ _ _ _ _ _ _ _ _ _ w850 _ _ _ _ _ _ _ _]
              tunnel: w140 -> [w181 w282 w331 w594 w616 w639 w663 w686 w711 w730 _ _ _ _ _ _ w872 w937 _ _ _ _ _ _ _]
              tunnel: [w183 w285 w338 w596 w619 w644 w667 w692 w716 w736 w751 w765 w771 w791 w799 w829 w835 w952 w969 w979 w990 w1001 w1012 w1020 w1037] -> w138
              tunnel: w139 -> [w183 w285 w338 w596 w619 w644 w667 w692 w716 w736 w751 w757 w778 w791 w799 w829 w835 w952 w969 w979 w990 w1001 w1012 w1025 w1037]
              tunnel: [w157 w284 w336 w595 w618 w643 w666 w691 w715 w735 w750 w766 w786 w790 w798 w828 w834 w914 w957 w976 w985 w997 w1008 w1023 w1039] -> w137
              tunnel: w136 -> [w157 w284 w336 w595 w618 w643 w666 w691 w715 w735 w750 w766 w786 w790 w798 w828 w834 w914 _ w975 w986 w998 w1009 w1023 w1039]
              tunnel: w135 -> [_ _ _ w586 w611 w634 w659 _ _ _ _ _ _ _ _ _ _ _ _ _ _ _ _ _ _]
              tunnel: w134 -> [_ _ _ w589 w614 _ _ _ _ _ _ _ _ _ _ _ _ _ _ _ _ _ _ _ _]
              tunnel: w133 -> [_ _ _ _ _ w636 w661 _ _ _ _ _ _ _ _ _ _ _ _ _ _ _ _ _ _]
              tunnel: w132 -> [_ _ _ _ _ _ _ w683 w707 _ _ _ _ _ _ _ _ _ _ _ _ _ _ _ _]
              tunnel: w131 -> [_ _ _ _ _ _ _ w687 w710 _ _ _ _ _ _ _ _ _ _ _ _ _ _ _ _]
              event Timeout {
                w168 = 2
                # "By default when clicking the RUN button, the camera will automatically stream images in secquence. After changing any of the instrument parameters, the VI will jump back to \"CMOS live\" state and into the \"Timeout\" event."
                n52 = event-data() -> ()  [unwired: 1 in, 3 out]
                n53 = Unbundle(w181) -> ("Device Z"=w171:refnum<k24>, "Device X"=w170:refnum<k24>, "Device Y"=w169:refnum<k24>)
                n54 = Unbundle By Name(w157) -> ("Laser X"=w165:dbl, "Laser Y"=w164:dbl)
                n55 = Unbundle By Name("Box") -> ("Width"=w159:dbl, "Height"=w158:dbl)
                n56 = Quotient & Remainder(x=w187, y=10) -> (x-y*floor(x/y)=w197:i32)  [unwired: 1 out]
                n57 = invoke class="KCubeDCServo" method="GetPositionCounter"(reference=w171) -> ("GetPositionCounter"=w180:i32)  [unwired: 2 in, 2 out]
                n58 = invoke class="KCubeDCServo" method="GetPositionCounter"(reference=w170) -> ("GetPositionCounter"=w179:i32)  [unwired: 2 in, 2 out]
                n59 = invoke class="KCubeDCServo" method="GetPositionCounter"(reference=w169) -> ("GetPositionCounter"=w178:i32)  [unwired: 2 in, 2 out]
                n60 = Quotient & Remainder(x=w187, y=5) -> (x-y*floor(x/y)=w200:i32)  [unwired: 1 out]
                n61 = Equal To 0?(x=w197) -> (x = 0?=w195:bool)
                n62 = Equal To 0?(x=w200) -> (x = 0?=w199:bool)
                n63 = Divide(x=w159, y=w168) -> (x/y=w163:dbl)
                n64 = Subtract(x=w165, y=w163) -> (x-y=w161:dbl)
                n65 = Divide(x=w158, y=w168) -> (x/y=w162:dbl)
                n66 = flat-sequence {
                  tunnel: [w252] -> w201
                  tunnel: w188 -> [w253]
                  tunnel: w190 -> [w251]
                  tunnel: [w250] -> w189
                  tunnel: w201 -> [w268]
                  tunnel: w186 -> [w267]
                  tunnel: w185 -> [w259]
                  tunnel: w157 -> [w255]
                  tunnel: w154 -> [w254]
                  frame #0 {
                    n67 = call "GetActImgMem.vi"("error in"=w251, "Camera Handle In"=w253) -> ("error out"=w250:errorcluster, "Image Memory Out"=w252:u8[])  [unwired: 6 in, 2 out]
                  }
                  frame #1 {
                    # "Display Image"
                    n68 = Unbundle(w267) -> ("Height"=w266:i32, "Width"=w265:i32)
                    n69 = Reshape Array(w268, w266, w265) -> (w264:u8[][])
                    n70 = call <vilib>:"Flatten Pixmap.vi"("colors"=u32[] [0, 65793, 131586, 197379, 263172, 328965, 394758, 460551, 526344, 592137, 657930, 723723, 789516, 855309, 921102, 986895, 1052688, 1118481, 1184274, 1250067, 1315860, 1381653, 1447446, 1513239, 1579032, 1644825, 1710618, 1776411, 1842204, 1907997, 1973790, 2039583, 2105376, 2171169, 2236962, 2302755, 2368548, 2434341, 2500134, 2565927, 2631720, 2697513, 2763306, 2829099, 2894892, 2960685, 3026478, 3092271, 3158064, 3223857, 3289650, 3355443, 3421236, 3487029, 3552822, 3618615, 3684408, 3750201, 3815994, 3881787, 3947580, 4013373, 4079166, 4144959, 4210752, 4276545, 4342338, 4408131, 4473924, 4539717, 4605510, 4671303, 4737096, 4802889, 4868682, 4934475, 5000268, 5066061, 5131854, 5197647, 5263440, 5329233, 5395026, 5460819, 5526612, 5592405, 5658198, 5723991, 5789784, 5855577, 5921370, 5987163, 6052956, 6118749, 6184542, 6250335, 6316128, 6381921, 6447714, 6513507, 6579300, 6645093, 6710886, 6776679, 6842472, 6908265, 6974058, 7039851, 7105644, 7171437, 7237230, 7303023, 7368816, 7434609, 7500402, 7566195, 7631988, 7697781, 7763574, 7829367, 7895160, 7960953, 8026746, 8092539, 8158332, 8224125, 8289918, 8355711, 8421504, 8487297, 8553090, 8618883, 8684676, 8750469, 8816262, 8882055, 8947848, 9013641, 9079434, 9145227, 9211020, 9276813, 9342606, 9408399, 9474192, 9539985, 9605778, 9671571, 9737364, 9803157, 9868950, 9934743, 10000536, 10066329, 10132122, 10197915, 10263708, 10329501, 10395294, 10461087, 10526880, 10592673, 10658466, 10724259, 10790052, 10855845, 10921638, 10987431, 11053224, 11119017, 11184810, 11250603, 11316396, 11382189, 11447982, 11513775, 11579568, 11645361, 11711154, 11776947, 11842740, 11908533, 11974326, 12040119, 12105912, 12171705, 12237498, 12303291, 12369084, 12434877, 12500670, 12566463, 12632256, 12698049, 12763842, 12829635, 12895428, 12961221, 13027014, 13092807, 13158600, 13224393, 13290186, 13355979, 13421772, 13487565, 13553358, 13619151, 13684944, 13750737, 13816530, 13882323, 13948116, 14013909, 14079702, 14145495, 14211288, 14277081, 14342874, 14408667, 14474460, 14540253, 14606046, 14671839, 14737632, 14803425, 14869218, 14935011, 15000804, 15066597, 15132390, 15198183, 15263976, 15329769, 15395562, 15461355, 15527148, 15592941, 15658734, 15724527, 15790320, 15856113, 15921906, 15987699, 16053492, 16119285, 16185078, 16250871, 16316664, 16382457, 16448250, 16514043, 16579836, 16645629, 16711422, 0] ("output array 2"), "8-bit pixmap"=w264) -> ("image data"=w263:T30)  [unwired: 9 in]
                    n71 = call <vilib>:"Draw Flattened Pixmap.vi"("image data"=w263) -> ("new picture"=w260:picture)  [unwired: 8 in]
                    n72 = call <vilib>:"Draw Rectangle.vi"("picture"=w260, "rect"=w259, "color(black)"=u32 16318226) -> ("new picture"=w258:picture)  [unwired: 6 in]
                    n73 = local read "Boolean"() -> (w256:bool)
                    n74 = case shown="True" w256 {
                      tunnel: w258 -> [w269 w272]
                      tunnel: [w269 w275] -> w257
                      tunnel: w255 -> [_ w274]
                      tunnel: w254 -> [_ w273]
                      frame False {
                      }
                      frame True {
                        n75 = call <vilib>:"Draw Rectangle.vi"("picture"=w272, "rect"=w273, "color(black)"=u32 6618880) -> ("new picture"=w271:picture)  [unwired: 6 in]
                        n76 = To Word Integer(number=w274) -> (16bit integer=w276:cluster{"Laser X":i16, "Laser Y":i16})
                        n77 = call <vilib>:"Draw Point.vi"("picture"=w271, "point(x,y)"=w276, "color(black)"=u32 16711680, "pen"=T25 {"Width"=5, "Style"=enum."Solid"}) -> ("new picture"=w275:picture)  [unwired: 5 in]
                      }
                    }
                    "Live video" <- w257
                  }
                }
                n78 = Subtract(x=w164, y=w162) -> (x-y=w160:dbl)
                n79 = Add(x=w162, y=w164) -> (x+y=w166:dbl)
                n80 = Add(x=w165, y=w163) -> (x+y=w167:dbl)
                n81 = Divide(x=w180, y=34304) -> (x/y=→"Z_axis":dbl)
                n82 = Divide(x=w179, y=34304) -> (x/y=→"X_axis":dbl)
                n83 = Divide(x=w178, y=34304) -> (x/y=→"Y_axis":dbl)
                n84 = Bundle By Name(cluster=T19 {"left"=0, "top"=0, "right"=0, "bottom"=0} ("rect"), "left"=w161, "top"=w160, "right"=w167, "bottom"=w166) -> (w154:T19)
                n85 = case shown="True" w199 {
                  tunnel: w188 -> [_ w236]
                  frame False {
                  }
                  frame True {
                    # "Set Slider Range"
                    n86 = call "GetFramesPerSecond.vi"("Camera Handle In"=w236) -> ("FPS"=→"FPS":dbl)  [unwired: 8 in, 2 out]
                    n87 = call "GetExposureRange.vi"("Camera Handle In"=w236) -> ("max"=w246:dbl, "min"=w247:dbl, "intervall"=w245:dbl)  [unwired: 6 in, 2 out]
                    n88 = Bundle("min"=w247, "max"=w246, "intervall"=w245) -> (w248:cluster{"min":dbl, "max":dbl, "intervall":dbl})  [unwired: 1 in]
                    n89 = property on="Exposure time (ms)" class="Schieberegler (strikt)"("Scale.Minimum"=w247, "Scale.Maximum"=w246, "Scale.Increment"=w245) -> ()  [unwired: 2 in, 2 out]
                    n90 = property on="Exposure time (ms)" class="Schieberegler (strikt)"("Data Range"=w248) -> ()  [unwired: 2 in, 2 out]
                    n91 = call "GetFrameTimeRange.vi"("Camera Handle In"=w236) -> ("max"=w242:dbl, "min"=w241:dbl, "interval"=w238:dbl)  [unwired: 6 in, 2 out]
                    n92 = Reciprocal(x=w242) -> (1/x=w240:dbl)
                    n93 = Reciprocal(x=w241) -> (1/x=w239:dbl)
                    n94 = property on="Frame rate" class="Schieberegler (strikt)"("Minimum"=w240, "Maximum"=w239, "Increment"=w238) -> ()  [unwired: 2 in, 2 out]
                    n95 = property on="Frame rate" class="Schieberegler (strikt)"("Scale.Minimum"=w240, "Scale.Maximum"=w239, "Scale.Increment"=w238) -> ()  [unwired: 2 in, 2 out]
                    n96 = call "GetPixelClockRange.vi"("Camera Handle In"=w236) -> ("Max"=w244:i32, "Min"=w243:i32)  [unwired: 7 in, 2 out]
                    n97 = property on="Pixel clock" class="Schieberegler (strikt)"("Scale.Minimum"=w243, "Scale.Maximum"=w244) -> ()  [unwired: 2 in, 2 out]
                    n98 = property on="Pixel clock" class="Schieberegler (strikt)"("Minimum"=w243, "Maximum"=w244) -> ()  [unwired: 2 in, 2 out]
                    n99 = call "SetAOI.vi"("Camera Handle In"=w236, "Mode"=32771) -> ("Width Out"=→"Width":i32, "Height Out"=→"Height":i32)  [unwired: 8 in, 4 out]
                  }
                }
                n100 = case shown="True" w195 {
                  tunnel: w188 -> [_ w205]
                  frame False {
                  }
                  frame True {
                    # "Set Exposure time, Pixelclock\nand Framerate"
                    n101 = call "ThorSetExposureTime.vi"("Mode"=u16 32900, "Exposure Time"="Exposure time (ms)", "Camera Handle In"=w205) -> ()  [unwired: 6 in, 3 out]
                    n102 = call "SetFrameRate.vi"("FPS"="Frame rate", "Camera Handle In"=w205) -> ()  [unwired: 7 in, 3 out]
                    n103 = call "SetPixelClock.vi"("Mode"=32770, "Pixel Clock"="Pixel clock", "Camera Handle In"=w205) -> ()  [unwired: 6 in, 3 out]
                    n104 = call "SetAutoParameter.vi"("enable"="Autogain", "Param"=34816, "Camera Handle In"=w205) -> ("Camera Handle Out"=w213:u32)  [unwired: 6 in, 2 out]
                    n105 = case shown="False" "Autogain" {
                      tunnel: w213 -> [w229 w232]
                      frame False {
                        # "Set Master Gain"
                        n106 = call "SetHardwareGain.vi"("Master Gain"="Master Gain", "Camera Handle In"=w229) -> ()  [unwired: 7 in, 3 out]
                      }
                      frame True {
                        w231 = 32768 items=["IS_GET_MASTER_GAIN"=32768]
                        # "On active AutoGain\nset Master Gain Slider Value"
                        n107 = call "SetHardwareGain.vi"("Mode"=w231, "Camera Handle In"=w232) -> ("Value"=w233:i32)  [unwired: 7 in, 2 out]
                        n108 = property on="Master Gain" class="Slide (strict)"("Value"=w233) -> ()  [unwired: 2 in, 2 out]
                      }
                    }
                    n109 = case shown="False" "Hotpixel correction 2" {
                      tunnel: w205 -> [w226 w228]
                      frame False {
                        n110 = call "SetHotPixelCorrection.vi"("Mode"=0, "Camera Handle In"=w226) -> ()  [unwired: 7 in, 3 out]
                      }
                      frame True {
                        n111 = call "SetHotPixelCorrection.vi"("Mode"=2, "Camera Handle In"=w228) -> ()  [unwired: 7 in, 3 out]
                      }
                    }
                    n112 = case shown="True" "Blacklevel compensation" {
                      tunnel: w205 -> [w221 w224]
                      tunnel: "Blacklevel Offset" -> [w219 w222]
                      frame False {
                        n113 = call "SetBlCompensation.vi"("Mode"=0, "offset"=w219, "Camera Handle In"=w221) -> ()  [unwired: 6 in, 3 out]
                      }
                      frame True {
                        n114 = call "SetBlCompensation.vi"("Mode"=1, "offset"=w222, "Camera Handle In"=w224) -> ()  [unwired: 6 in, 3 out]
                      }
                    }
                    n115 = case shown="True" "Edge Filter Enable / Disable" {
                      tunnel: w205 -> [w215 w218]
                      frame False {
                        n116 = call "SetEdgeEnhancement.vi"("Mode"=0, "Camera Handle In"=w215) -> ()  [unwired: 8 in, 2 out]
                      }
                      frame True {
                        n117 = call "SetEdgeEnhancement.vi"("Mode"="Edge Filter", "Camera Handle In"=w218) -> ()  [unwired: 8 in, 2 out]
                      }
                    }
                  }
                }
                n118 = local read "Frame rate"() -> (w194:dbl)
                n119 = Reciprocal(x=w194) -> (1/x=w193:dbl)
                n120 = Multiply(x=w193, y=1000) -> (x*y=w191:dbl)
                n121 = Wait Until Next ms Multiple(millisecond multiple=w191) -> ()  [unwired: 1 out]
              }
              event "Reset": Value Change {
                n122 = event-data() -> ()  [unwired: 1 in, 6 out]
                n123 = Unbundle(w282) -> ("Device Z"=w281:refnum<k24>, "Device X"=w280:refnum<k24>, "Device Y"=w279:refnum<k24>)
                n124 = stacked-sequence {
                  tunnel: w281 -> [w292 _ _ _ _ w314 w319 w322 _]
                  tunnel: w279 -> [_ _ w298 _ w310 _ _ w321 _]
                  tunnel: w280 -> [_ w294 _ w305 _ _ _ w320 _]
                  frame #0 {
                    # "Move Z to maxinum"
                    n125 = invoke class="KCubeDCServo" method="MoveTo"(reference=w292, "position"=12.0, "waitTimeout"=0) -> ()  [unwired: 2 in, 5 out]
                    n126 = Wait (ms)(milliseconds to wait=u32 10000) -> ()  [unwired: 1 out]
                  }
                  frame #1 {
                    # "Make X home"
                    n127 = invoke class="KCubeDCServo" method="Home"(reference=w294, "waitTimeout"=0) -> (reference out=w293:refnum<k24>)  [unwired: 2 in, 3 out]
                    n128 = invoke class="KCubeDCServo" method="ClearDeviceExceptions"(reference=w293) -> ()  [unwired: 2 in, 3 out]
                    n129 = Wait (ms)(milliseconds to wait=u32 30000) -> ()  [unwired: 1 out]
                  }
                  frame #2 {
                    # "Make Y home"
                    n130 = invoke class="KCubeDCServo" method="Home"(reference=w298, "waitTimeout"=0) -> (reference out=w297:refnum<k24>)  [unwired: 2 in, 3 out]
                    n131 = invoke class="KCubeDCServo" method="ClearDeviceExceptions"(reference=w297) -> ()  [unwired: 2 in, 3 out]
                    n132 = Wait (ms)(milliseconds to wait=u32 30000) -> ()  [unwired: 1 out]
                  }
                  frame #3 {
                    # "Move X to center"
                    n133 = invoke class="KCubeDCServo" method="MoveTo"(reference=w305, "position"=7.0, "waitTimeout"=0) -> (reference out=w301:refnum<k24>)  [unwired: 2 in, 4 out]
                    n134 = invoke class="KCubeDCServo" method="ClearDeviceExceptions"(reference=w301) -> ()  [unwired: 2 in, 3 out]
                    n135 = Wait (ms)(milliseconds to wait=u32 5000) -> ()  [unwired: 1 out]
                  }
                  frame #4 {
                    # "Move Y to center"
                    n136 = invoke class="KCubeDCServo" method="MoveTo"(reference=w310, "position"=7.0, "waitTimeout"=0) -> (reference out=w306:refnum<k24>)  [unwired: 2 in, 4 out]
                    n137 = invoke class="KCubeDCServo" method="ClearDeviceExceptions"(reference=w306) -> ()  [unwired: 2 in, 3 out]
                    n138 = Wait (ms)(milliseconds to wait=u32 5000) -> ()  [unwired: 1 out]
                  }
                  frame #5 {
                    # "Z: home"
                    n139 = invoke class="KCubeDCServo" method="Home"(reference=w314, "waitTimeout"=0) -> (reference out=w311:refnum<k24>)  [unwired: 2 in, 3 out]
                    n140 = invoke class="KCubeDCServo" method="ClearDeviceExceptions"(reference=w311) -> ()  [unwired: 2 in, 3 out]
                    n141 = Wait (ms)(milliseconds to wait=u32 40000) -> ()  [unwired: 1 out]
                  }
                  frame #6 {
                    # "Move satge along Z about 0.5mm"
                    n142 = invoke class="KCubeDCServo" method="MoveTo"(reference=w319, "position"=4.5, "waitTimeout"=0) -> (reference out=w315:refnum<k24>)  [unwired: 2 in, 4 out]
                    n143 = Wait (ms)(milliseconds to wait=u32 5000) -> ()  [unwired: 1 out]
                    n144 = invoke class="KCubeDCServo" method="ClearDeviceExceptions"(reference=w315) -> ()  [unwired: 2 in, 3 out]
                  }
                  frame #7 {
                    n145 = invoke class="KCubeDCServo" method="ClearDeviceExceptions"(reference=w320) -> ()  [unwired: 2 in, 3 out]
                    n146 = invoke class="KCubeDCServo" method="ClearDeviceExceptions"(reference=w321) -> ()  [unwired: 2 in, 3 out]
                    n147 = invoke class="KCubeDCServo" method="ClearDeviceExceptions"(reference=w322) -> ()  [unwired: 2 in, 3 out]
                  }
                  frame #8 {
                    n148 = call "Display Message to User"("Enable"=TRUE, "Message"="Reset has been completed!!") -> ()  [unwired: 8 in, 2 out]
                  }
                }
              }
              event "Scan": Value Change {
                n149 = event-data() -> ()  [unwired: 1 in, 6 out]
                n150 = Unbundle By Name(w325) -> ("left"=w335:i16, "top"=w333:i16, "right"=w334:i16, "bottom"=w332:i16)
                n151 = stacked-sequence {
                  tunnel: w336 -> [_ w372 _ _]
                  tunnel: w335 -> [_ w354 w405 _]
                  tunnel: w334 -> [_ _ w406 _]
                  tunnel: w333 -> [_ w353 w398 _]
                  tunnel: w332 -> [_ _ w399 _]
                  tunnel: w331 -> [_ w357 w397 _]
                  tunnel: w330 -> [_ w356 _ _]
                  tunnel: [_ w355 _ _] -> w329
                  tunnel: w328 -> [w340 _ w396 _]
                  tunnel: w327 -> [w341 _ w395 _]
                  tunnel: "Save Path" -> [w343 _ w394 _]
                  frame #0 {
                    n152 = Unbundle(w341) -> ("Height"=w346:i32, "Width"=w345:i32)
                    n153 = Build Path(base path=w343, name or relative path="Crop_Area.png") -> (appended path=w347:path)
                    n154 = call "GetActImgMem.vi"("Camera Handle In"=w340) -> ("Image Memory Out"=w350:u8[])  [unwired: 7 in, 3 out]
                    n155 = Reshape Array(w350, w346, w345) -> (w351:u8[][])
                    n156 = call <vilib>:"Flatten Pixmap.vi"("colors"=u32[] [0, 65793, 131586, 197379, 263172, 328965, 394758, 460551, 526344, 592137, 657930, 723723, 789516, 855309, 921102, 986895, 1052688, 1118481, 1184274, 1250067, 1315860, 1381653, 1447446, 1513239, 1579032, 1644825, 1710618, 1776411, 1842204, 1907997, 1973790, 2039583, 2105376, 2171169, 2236962, 2302755, 2368548, 2434341, 2500134, 2565927, 2631720, 2697513, 2763306, 2829099, 2894892, 2960685, 3026478, 3092271, 3158064, 3223857, 3289650, 3355443, 3421236, 3487029, 3552822, 3618615, 3684408, 3750201, 3815994, 3881787, 3947580, 4013373, 4079166, 4144959, 4210752, 4276545, 4342338, 4408131, 4473924, 4539717, 4605510, 4671303, 4737096, 4802889, 4868682, 4934475, 5000268, 5066061, 5131854, 5197647, 5263440, 5329233, 5395026, 5460819, 5526612, 5592405, 5658198, 5723991, 5789784, 5855577, 5921370, 5987163, 6052956, 6118749, 6184542, 6250335, 6316128, 6381921, 6447714, 6513507, 6579300, 6645093, 6710886, 6776679, 6842472, 6908265, 6974058, 7039851, 7105644, 7171437, 7237230, 7303023, 7368816, 7434609, 7500402, 7566195, 7631988, 7697781, 7763574, 7829367, 7895160, 7960953, 8026746, 8092539, 8158332, 8224125, 8289918, 8355711, 8421504, 8487297, 8553090, 8618883, 8684676, 8750469, 8816262, 8882055, 8947848, 9013641, 9079434, 9145227, 9211020, 9276813, 9342606, 9408399, 9474192, 9539985, 9605778, 9671571, 9737364, 9803157, 9868950, 9934743, 10000536, 10066329, 10132122, 10197915, 10263708, 10329501, 10395294, 10461087, 10526880, 10592673, 10658466, 10724259, 10790052, 10855845, 10921638, 10987431, 11053224, 11119017, 11184810, 11250603, 11316396, 11382189, 11447982, 11513775, 11579568, 11645361, 11711154, 11776947, 11842740, 11908533, 11974326, 12040119, 12105912, 12171705, 12237498, 12303291, 12369084, 12434877, 12500670, 12566463, 12632256, 12698049, 12763842, 12829635, 12895428, 12961221, 13027014, 13092807, 13158600, 13224393, 13290186, 13355979, 13421772, 13487565, 13553358, 13619151, 13684944, 13750737, 13816530, 13882323, 13948116, 14013909, 14079702, 14145495, 14211288, 14277081, 14342874, 14408667, 14474460, 14540253, 14606046, 14671839, 14737632, 14803425, 14869218, 14935011, 15000804, 15066597, 15132390, 15198183, 15263976, 15329769, 15395562, 15461355, 15527148, 15592941, 15658734, 15724527, 15790320, 15856113, 15921906, 15987699, 16053492, 16119285, 16185078, 16250871, 16316664, 16382457, 16448250, 16514043, 16579836, 16645629, 16711422, 0] ("output array 2"), "8-bit pixmap"=w351) -> ("image data"=w348:T30)  [unwired: 9 in]
                    n157 = Wait (ms)(milliseconds to wait=u32 300) -> ()  [unwired: 1 out]
                    n158 = call <vilib>:"Write PNG File.vi"("image data"=w348, "path to PNG file"=w347) -> ()  [unwired: 8 in, 2 out]
                  }
                  frame #1 {
                    n159 = Unbundle By Name(w372) -> ("Laser X"=w364:dbl, "Laser Y"=w363:dbl)
                    n160 = Subtract(x=w364, y=w354) -> (x-y=w362:dbl)
                    n161 = Subtract(x=w363, y=w353) -> (x-y=w360:dbl)
                    n162 = Divide(x=0.0877, y=1000.0) -> (x/y=w361:dbl)
                    n163 = Multiply(x=w361, y=w362) -> (x*y=w359:dbl)
                    n164 = Multiply(x=w361, y=w360) -> (x*y=w358:dbl)
                    n165 = call "StageReadPos.vi"("error in (no error)"=w356, "Stage Select"=StageSelect."X axis", "Device In"=w357) -> ("error out"=w371:errorcluster, "CurrentPosition"=w369:dbl)  [unwired: 7 in]
                    n166 = call "StageReadPos.vi"("error in (no error)"=w356, "Stage Select"=StageSelect."Y axis", "Device In"=w357) -> ("error out"=w367:errorcluster, "CurrentPosition"=w366:dbl)  [unwired: 7 in]
                    n167 = stacked-sequence {
                      tunnel: w371 -> [w391 _]
                      tunnel: w369 -> [w389 _]
                      tunnel: [w387 _] -> w365
                      tunnel: w359 -> [w386 _]
                      tunnel: w357 -> [w385 _]
                      frame #0 {
                        n168 = Add(x=w386, y=w389) -> (x+y=w388:dbl)
                        n169 = call "StageToPos.vi"("error in (no error)"=w391, "Move to pos"=w388, "Stage Select"=StageSelect."X axis", "Device In"=w385) -> ("error out"=w387:errorcluster)  [unwired: 7 in]
                      }
                      frame #1 {
                        n170 = Wait (ms)(milliseconds to wait=u32 400) -> ()  [unwired: 1 out]
                      }
                    }
                    n171 = stacked-sequence {
                      tunnel: w367 -> [w382 _]
                      tunnel: w366 -> [w381 _]
                      tunnel: w365 -> [w379 _]
                      tunnel: w358 -> [w377 _]
                      tunnel: w357 -> [w376 _]
                      tunnel: [w375 _] -> w355
                      frame #0 {
                        n172 = Add(x=w377, y=w381) -> (x+y=w380:dbl)
                        n173 = call "StageToPos.vi"("error in (no error)"=w382, "Move to pos"=w380, "Stage Select"=StageSelect."Y axis", "Device In"=w376) -> ("error out"=w378:errorcluster)  [unwired: 7 in]
                        n174 = Merge Errors(w379, w378) -> (w375:errorcluster)
                      }
                      frame #1 {
                        n175 = Wait (ms)(milliseconds to wait=u32 400) -> ()  [unwired: 1 out]
                      }
                    }
                    n176 = Wait (ms)(milliseconds to wait=u32 100) -> ()  [unwired: 1 out]
                  }
                  frame #2 {
                    n177 = Subtract(x=w399, y=w398) -> (x-y=w401:i16)
                    n178 = Subtract(x=w406, y=w405) -> (x-y=w404:i16)
                    n179 = Divide(x=w401, y=i16 50) -> (x/y=w393:dbl)
                    n180 = Divide(x=w404, y=i16 50) -> (x/y=w402:dbl)
                    n181 = for {
                      N: w393 -> [w413]
                      tunnel: w402 -> [w407]
                      tunnel: w397 -> [w417]
                      tunnel: w396 -> [w416]
                      tunnel: w395 -> [w415]
                      tunnel: w394 -> [w414]
                      i -> [w410]
                      n182 = Round Toward -Infinity(1:w407) -> (0:→"Total_Frame_X":dbl)
                      n183 = Increment(x=w410) -> (x+1=→"Frame_Y":i32)
                      n184 = Divide(x=w410, y=2) -> (x/y=w422:dbl)
                      n185 = Round Toward -Infinity(1:w422) -> (0:w419:dbl)
                      n186 = Round Toward +Infinity(x=w422) -> (ceil(x): smallest int >= x=w420:dbl)
                      n187 = Equal?(x=w420, y=w419) -> (x = y?=w418:bool)
                      n188 = stacked-sequence {
                        tunnel: w418 -> [_ w435 w487]
                        tunnel: w407 -> [_ _ w486]
                        tunnel: w417 -> [w432 _ w485]
                        tunnel: w416 -> [_ w436 w484]
                        tunnel: w415 -> [_ w437 w483]
                        tunnel: w414 -> [_ w438 w482]
                        tunnel: w410 -> [_ w434 w481]
                        tunnel: w407 -> [_ w433 w480]
                        tunnel: [_ _ w479] -> w412
                        frame #0 {
                          w430 = 1 items=["Forward"=1, "Backward"=2] ("direction")
                          n189 = Unbundle By Name(w432) -> ("Device Y"=w431:refnum<k24>)  [unwired: 2 out]
                          n190 = Divide(x=0.0877 ("y"), y=1000.0) -> (x/y=w423:dbl)
                          n191 = Multiply(x=50.0, y=w423) -> (x*y=w426:dbl)
                          n192 = invoke class="KCubeDCServo" method="MoveRelative"(reference=w431, "direction"=w430, "stepSize"=w426, "waitTimeout"=0) -> ()  [unwired: 2 in, 6 out]
                          n193 = Wait (ms)(milliseconds to wait=u32 300) -> ()  [unwired: 1 out]
                        }
                        frame #1 {
                          n194 = case shown="False" w435 {
                            tunnel: w438 -> [w445 w464]
                            tunnel: w437 -> [w443 w463]
                            tunnel: w436 -> [w444 w462]
                            tunnel: w434 -> [w441 w460]
                            tunnel: w433 -> [w440 _]
                            frame False {
                              n195 = Round Toward -Infinity(1:w440) -> (0:w439:dbl)
                              n196 = Increment(x=w441) -> (x+1=w446:i32)
                              n197 = Number To Decimal String(number=w439) -> (decimal integer string=w442:string)  [unwired: 1 in]
                              n198 = Number To Decimal String(number=w446) -> (decimal integer string=w451:string)  [unwired: 1 in]
                              n199 = Concatenate Strings("x" ("string"), w442, "_y" ("string"), w451, ".png" ("string")) -> (w455:string)
                              n200 = Unbundle(w443) -> ("Height"=w449:i32, "Width"=w448:i32)
                              n201 = Build Path(base path=w445, name or relative path=w455) -> (appended path=w450:path)
                              n202 = call "GetActImgMem.vi"("Camera Handle In"=w444) -> ("Image Memory Out"=w458:u8[])  [unwired: 7 in, 3 out]
                              n203 = Reshape Array(w458, w449, w448) -> (w459:u8[][])
                              n204 = call <vilib>:"Flatten Pixmap.vi"("colors"=u32[] [0, 65793, 131586, 197379, 263172, 328965, 394758, 460551, 526344, 592137, 657930, 723723, 789516, 855309, 921102, 986895, 1052688, 1118481, 1184274, 1250067, 1315860, 1381653, 1447446, 1513239, 1579032, 1644825, 1710618, 1776411, 1842204, 1907997, 1973790, 2039583, 2105376, 2171169, 2236962, 2302755, 2368548, 2434341, 2500134, 2565927, 2631720, 2697513, 2763306, 2829099, 2894892, 2960685, 3026478, 3092271, 3158064, 3223857, 3289650, 3355443, 3421236, 3487029, 3552822, 3618615, 3684408, 3750201, 3815994, 3881787, 3947580, 4013373, 4079166, 4144959, 4210752, 4276545, 4342338, 4408131, 4473924, 4539717, 4605510, 4671303, 4737096, 4802889, 4868682, 4934475, 5000268, 5066061, 5131854, 5197647, 5263440, 5329233, 5395026, 5460819, 5526612, 5592405, 5658198, 5723991, 5789784, 5855577, 5921370, 5987163, 6052956, 6118749, 6184542, 6250335, 6316128, 6381921, 6447714, 6513507, 6579300, 6645093, 6710886, 6776679, 6842472, 6908265, 6974058, 7039851, 7105644, 7171437, 7237230, 7303023, 7368816, 7434609, 7500402, 7566195, 7631988, 7697781, 7763574, 7829367, 7895160, 7960953, 8026746, 8092539, 8158332, 8224125, 8289918, 8355711, 8421504, 8487297, 8553090, 8618883, 8684676, 8750469, 8816262, 8882055, 8947848, 9013641, 9079434, 9145227, 9211020, 9276813, 9342606, 9408399, 9474192, 9539985, 9605778, 9671571, 9737364, 9803157, 9868950, 9934743, 10000536, 10066329, 10132122, 10197915, 10263708, 10329501, 10395294, 10461087, 10526880, 10592673, 10658466, 10724259, 10790052, 10855845, 10921638, 10987431, 11053224, 11119017, 11184810, 11250603, 11316396, 11382189, 11447982, 11513775, 11579568, 11645361, 11711154, 11776947, 11842740, 11908533, 11974326, 12040119, 12105912, 12171705, 12237498, 12303291, 12369084, 12434877, 12500670, 12566463, 12632256, 12698049, 12763842, 12829635, 12895428, 12961221, 13027014, 13092807, 13158600, 13224393, 13290186, 13355979, 13421772, 13487565, 13553358, 13619151, 13684944, 13750737, 13816530, 13882323, 13948116, 14013909, 14079702, 14145495, 14211288, 14277081, 14342874, 14408667, 14474460, 14540253, 14606046, 14671839, 14737632, 14803425, 14869218, 14935011, 15000804, 15066597, 15132390, 15198183, 15263976, 15329769, 15395562, 15461355, 15527148, 15592941, 15658734, 15724527, 15790320, 15856113, 15921906, 15987699, 16053492, 16119285, 16185078, 16250871, 16316664, 16382457, 16448250, 16514043, 16579836, 16645629, 16711422, 0] ("output array 2"), "8-bit pixmap"=w459) -> ("image data"=w456:T30)  [unwired: 9 in]
                              n205 = Wait (ms)(milliseconds to wait=u32 300) -> ()  [unwired: 1 out]
                              n206 = call <vilib>:"Write PNG File.vi"("image data"=w456, "path to PNG file"=w450) -> ()  [unwired: 8 in, 2 out]
                            }
                            frame True {
                              n207 = Increment(x=w460) -> (x+1=w465:i32)
                              n208 = Number To Decimal String(number=w465) -> (decimal integer string=w470:string)  [unwired: 1 in]
                              n209 = Concatenate Strings("x" ("string"), "0" ("string"), "_y" ("string"), w470, ".png" ("string")) -> (w474:string)
                              n210 = Unbundle(w463) -> ("Height"=w468:i32, "Width"=w467:i32)
                              n211 = Build Path(base path=w464, name or relative path=w474) -> (appended path=w469:path)
                              n212 = call "GetActImgMem.vi"("Camera Handle In"=w462) -> ("Image Memory Out"=w477:u8[])  [unwired: 7 in, 3 out]
                              n213 = Reshape Array(w477, w468, w467) -> (w478:u8[][])
                              n214 = call <vilib>:"Flatten Pixmap.vi"("colors"=u32[] [0, 65793, 131586, 197379, 263172, 328965, 394758, 460551, 526344, 592137, 657930, 723723, 789516, 855309, 921102, 986895, 1052688, 1118481, 1184274, 1250067, 1315860, 1381653, 1447446, 1513239, 1579032, 1644825, 1710618, 1776411, 1842204, 1907997, 1973790, 2039583, 2105376, 2171169, 2236962, 2302755, 2368548, 2434341, 2500134, 2565927, 2631720, 2697513, 2763306, 2829099, 2894892, 2960685, 3026478, 3092271, 3158064, 3223857, 3289650, 3355443, 3421236, 3487029, 3552822, 3618615, 3684408, 3750201, 3815994, 3881787, 3947580, 4013373, 4079166, 4144959, 4210752, 4276545, 4342338, 4408131, 4473924, 4539717, 4605510, 4671303, 4737096, 4802889, 4868682, 4934475, 5000268, 5066061, 5131854, 5197647, 5263440, 5329233, 5395026, 5460819, 5526612, 5592405, 5658198, 5723991, 5789784, 5855577, 5921370, 5987163, 6052956, 6118749, 6184542, 6250335, 6316128, 6381921, 6447714, 6513507, 6579300, 6645093, 6710886, 6776679, 6842472, 6908265, 6974058, 7039851, 7105644, 7171437, 7237230, 7303023, 7368816, 7434609, 7500402, 7566195, 7631988, 7697781, 7763574, 7829367, 7895160, 7960953, 8026746, 8092539, 8158332, 8224125, 8289918, 8355711, 8421504, 8487297, 8553090, 8618883, 8684676, 8750469, 8816262, 8882055, 8947848, 9013641, 9079434, 9145227, 9211020, 9276813, 9342606, 9408399, 9474192, 9539985, 9605778, 9671571, 9737364, 9803157, 9868950, 9934743, 10000536, 10066329, 10132122, 10197915, 10263708, 10329501, 10395294, 10461087, 10526880, 10592673, 10658466, 10724259, 10790052, 10855845, 10921638, 10987431, 11053224, 11119017, 11184810, 11250603, 11316396, 11382189, 11447982, 11513775, 11579568, 11645361, 11711154, 11776947, 11842740, 11908533, 11974326, 12040119, 12105912, 12171705, 12237498, 12303291, 12369084, 12434877, 12500670, 12566463, 12632256, 12698049, 12763842, 12829635, 12895428, 12961221, 13027014, 13092807, 13158600, 13224393, 13290186, 13355979, 13421772, 13487565, 13553358, 13619151, 13684944, 13750737, 13816530, 13882323, 13948116, 14013909, 14079702, 14145495, 14211288, 14277081, 14342874, 14408667, 14474460, 14540253, 14606046, 14671839, 14737632, 14803425, 14869218, 14935011, 15000804, 15066597, 15132390, 15198183, 15263976, 15329769, 15395562, 15461355, 15527148, 15592941, 15658734, 15724527, 15790320, 15856113, 15921906, 15987699, 16053492, 16119285, 16185078, 16250871, 16316664, 16382457, 16448250, 16514043, 16579836, 16645629, 16711422, 0] ("output array 2"), "8-bit pixmap"=w478) -> ("image data"=w475:T30)  [unwired: 9 in]
                              n215 = Wait (ms)(milliseconds to wait=u32 300) -> ()  [unwired: 1 out]
                              n216 = call <vilib>:"Write PNG File.vi"("image data"=w475, "path to PNG file"=w469) -> ()  [unwired: 8 in, 2 out]
                            }
                          }
                        }
                        frame #2 {
                          n217 = case shown="False" w487 {
                            tunnel: w486 -> [w495 w544]
                            tunnel: w485 -> [w494 w543]
                            tunnel: w484 -> [w492 w542]
                            tunnel: w483 -> [w489 w541]
                            tunnel: w482 -> [w493 w540]
                            tunnel: w481 -> [w491 w539]
                            tunnel: w480 -> [w490 _]
                            tunnel: [w488 w538] -> w479
                            frame False {
                              n218 = for {
                                N: w495 -> [_]
                                tunnel: w494 -> [w502]
                                tunnel: w493 -> [w501]
                                tunnel: w492 -> [w500]
                                tunnel: w491 -> [w499]
                                tunnel: w490 -> [w498]
                                tunnel: w489 -> [w497]
                                tunnel: [w496] -> w488
                                i -> [w496]
                                n219 = stacked-sequence {
                                tunnel: w502 -> [_ w507 _]
                                tunnel: w501 -> [_ _ w526]
                                tunnel: w500 -> [_ _ w525]
                                tunnel: w499 -> [_ _ w520]
                                tunnel: w496 -> [_ _ w518]
                                tunnel: w498 -> [_ _ w517]
                                tunnel: w497 -> [_ _ w524]
                                frame #0 {
                                n220 = Wait (ms)(milliseconds to wait=u32 100) -> ()  [unwired: 1 out]
                                }
                                frame #1 {
                                w513 = 2 items=["Forward"=1, "Backward"=2] ("direction")
                                n221 = Unbundle By Name(w507) -> ("Device X"=w508:refnum<k24>)  [unwired: 2 out]
                                n222 = Divide(x=0.0877 ("y"), y=1000.0) -> (x/y=w505:dbl)
                                n223 = Multiply(x=50.0, y=w505) -> (x*y=w509:dbl)
                                n224 = invoke class="KCubeDCServo" method="MoveRelative"(reference=w508, "direction"=w513, "stepSize"=w509, "waitTimeout"=0) -> ()  [unwired: 2 in, 6 out]
                                n225 = Wait (ms)(milliseconds to wait=u32 450) -> ()  [unwired: 1 out]
                                }
                                frame #2 {
                                n226 = Round Toward -Infinity(1:w517) -> (0:w516:dbl)
                                n227 = Decrement(x=w516) -> (x-1=w515:dbl)
                                n228 = Subtract(x=w515, y=w518) -> (x-y=w514:dbl)
                                n229 = Increment(x=w520) -> (x+1=w519:i32)
                                n230 = Number To Decimal String(number=w514) -> (decimal integer string=w529:string)  [unwired: 1 in]
                                n231 = Number To Decimal String(number=w519) -> (decimal integer string=w528:string)  [unwired: 1 in]
                                n232 = Concatenate Strings("x" ("string"), w529, "_y" ("string"), w528, ".png" ("string")) -> (w533:string)
                                n233 = Unbundle(w524) -> ("Height"=w523:i32, "Width"=w522:i32)
                                n234 = Build Path(base path=w526, name or relative path=w533) -> (appended path=w527:path)
                                n235 = call "GetActImgMem.vi"("Camera Handle In"=w525) -> ("Image Memory Out"=w536:u8[])  [unwired: 7 in, 3 out]
                                n236 = Reshape Array(w536, w523, w522) -> (w537:u8[][])
                                n237 = call <vilib>:"Flatten Pixmap.vi"("colors"=u32[] [0, 65793, 131586, 197379, 263172, 328965, 394758, 460551, 526344, 592137, 657930, 723723, 789516, 855309, 921102, 986895, 1052688, 1118481, 1184274, 1250067, 1315860, 1381653, 1447446, 1513239, 1579032, 1644825, 1710618, 1776411, 1842204, 1907997, 1973790, 2039583, 2105376, 2171169, 2236962, 2302755, 2368548, 2434341, 2500134, 2565927, 2631720, 2697513, 2763306, 2829099, 2894892, 2960685, 3026478, 3092271, 3158064, 3223857, 3289650, 3355443, 3421236, 3487029, 3552822, 3618615, 3684408, 3750201, 3815994, 3881787, 3947580, 4013373, 4079166, 4144959, 4210752, 4276545, 4342338, 4408131, 4473924, 4539717, 4605510, 4671303, 4737096, 4802889, 4868682, 4934475, 5000268, 5066061, 5131854, 5197647, 5263440, 5329233, 5395026, 5460819, 5526612, 5592405, 5658198, 5723991, 5789784, 5855577, 5921370, 5987163, 6052956, 6118749, 6184542, 6250335, 6316128, 6381921, 6447714, 6513507, 6579300, 6645093, 6710886, 6776679, 6842472, 6908265, 6974058, 7039851, 7105644, 7171437, 7237230, 7303023, 7368816, 7434609, 7500402, 7566195, 7631988, 7697781, 7763574, 7829367, 7895160, 7960953, 8026746, 8092539, 8158332, 8224125, 8289918, 8355711, 8421504, 8487297, 8553090, 8618883, 8684676, 8750469, 8816262, 8882055, 8947848, 9013641, 9079434, 9145227, 9211020, 9276813, 9342606, 9408399, 9474192, 9539985, 9605778, 9671571, 9737364, 9803157, 9868950, 9934743, 10000536, 10066329, 10132122, 10197915, 10263708, 10329501, 10395294, 10461087, 10526880, 10592673, 10658466, 10724259, 10790052, 10855845, 10921638, 10987431, 11053224, 11119017, 11184810, 11250603, 11316396, 11382189, 11447982, 11513775, 11579568, 11645361, 11711154, 11776947, 11842740, 11908533, 11974326, 12040119, 12105912, 12171705, 12237498, 12303291, 12369084, 12434877, 12500670, 12566463, 12632256, 12698049, 12763842, 12829635, 12895428, 12961221, 13027014, 13092807, 13158600, 13224393, 13290186, 13355979, 13421772, 13487565, 13553358, 13619151, 13684944, 13750737, 13816530, 13882323, 13948116, 14013909, 14079702, 14145495, 14211288, 14277081, 14342874, 14408667, 14474460, 14540253, 14606046, 14671839, 14737632, 14803425, 14869218, 14935011, 15000804, 15066597, 15132390, 15198183, 15263976, 15329769, 15395562, 15461355, 15527148, 15592941, 15658734, 15724527, 15790320, 15856113, 15921906, 15987699, 16053492, 16119285, 16185078, 16250871, 16316664, 16382457, 16448250, 16514043, 16579836, 16645629, 16711422, 0] ("output array 2"), "8-bit pixmap"=w537) -> ("image data"=w534:T30)  [unwired: 9 in]
                                n238 = Wait (ms)(milliseconds to wait=u32 300) -> ()  [unwired: 1 out]
                                n239 = call <vilib>:"Write PNG File.vi"("image data"=w534, "path to PNG file"=w527) -> ()  [unwired: 8 in, 2 out]
                                }
                                }
                              }
                            }
                            frame True {
                              n240 = for {
                                N: w544 -> [_]
                                tunnel: w543 -> [w550]
                                tunnel: w542 -> [w549]
                                tunnel: w541 -> [w548]
                                tunnel: w540 -> [w547]
                                tunnel: w539 -> [w546]
                                tunnel: [w545] -> w538
                                i -> [w545]
                                n241 = stacked-sequence {
                                tunnel: w550 -> [_ w556 _]
                                tunnel: w549 -> [_ _ w576]
                                tunnel: w548 -> [_ _ w575]
                                tunnel: w547 -> [_ _ w573]
                                tunnel: w545 -> [_ _ w563]
                                tunnel: w546 -> [_ _ w565]
                                frame #0 {
                                n242 = Wait (ms)(milliseconds to wait=u32 100) -> ()  [unwired: 1 out]
                                }
                                frame #1 {
                                w561 = 1 items=["Forward"=1, "Backward"=2] ("direction")
                                n243 = Unbundle By Name(w556) -> ("Device X"=w555:refnum<k24>)  [unwired: 2 out]
                                n244 = Divide(x=0.0877 ("y"), y=1000.0) -> (x/y=w552:dbl)
                                n245 = Multiply(x=50.0, y=w552) -> (x*y=w557:dbl)
                                n246 = invoke class="KCubeDCServo" method="MoveRelative"(reference=w555, "direction"=w561, "stepSize"=w557, "waitTimeout"=0) -> ()  [unwired: 2 in, 6 out]
                                n247 = Wait (ms)(milliseconds to wait=u32 400) -> ()  [unwired: 1 out]
                                }
                                frame #2 {
                                n248 = Increment(x=w563) -> (x+1=w562:i32)
                                n249 = Increment(x=w565) -> (x+1=w564:i32)
                                n250 = Number To Decimal String(number=w564) -> (decimal integer string=w568:string)  [unwired: 1 in]
                                n251 = Number To Decimal String(number=w562) -> (decimal integer string=w569:string)  [unwired: 1 in]
                                n252 = Concatenate Strings("x" ("string"), w569, "_y" ("string"), w568, ".png" ("string")) -> (w574:string)
                                n253 = Build Path(base path=w573, name or relative path=w574) -> (appended path=w567:path)
                                n254 = call "GetActImgMem.vi"("Camera Handle In"=w576) -> ("Image Memory Out"=w579:u8[])  [unwired: 7 in, 3 out]
                                n255 = Unbundle(w575) -> ("Height"=w580:i32, "Width"=w581:i32)
                                n256 = Reshape Array(w579, w580, w581) -> (w582:u8[][])
                                n257 = call <vilib>:"Flatten Pixmap.vi"("colors"=u32[] [0, 65793, 131586, 197379, 263172, 328965, 394758, 460551, 526344, 592137, 657930, 723723, 789516, 855309, 921102, 986895, 1052688, 1118481, 1184274, 1250067, 1315860, 1381653, 1447446, 1513239, 1579032, 1644825, 1710618, 1776411, 1842204, 1907997, 1973790, 2039583, 2105376, 2171169, 2236962, 2302755, 2368548, 2434341, 2500134, 2565927, 2631720, 2697513, 2763306, 2829099, 2894892, 2960685, 3026478, 3092271, 3158064, 3223857, 3289650, 3355443, 3421236, 3487029, 3552822, 3618615, 3684408, 3750201, 3815994, 3881787, 3947580, 4013373, 4079166, 4144959, 4210752, 4276545, 4342338, 4408131, 4473924, 4539717, 4605510, 4671303, 4737096, 4802889, 4868682, 4934475, 5000268, 5066061, 5131854, 5197647, 5263440, 5329233, 5395026, 5460819, 5526612, 5592405, 5658198, 5723991, 5789784, 5855577, 5921370, 5987163, 6052956, 6118749, 6184542, 6250335, 6316128, 6381921, 6447714, 6513507, 6579300, 6645093, 6710886, 6776679, 6842472, 6908265, 6974058, 7039851, 7105644, 7171437, 7237230, 7303023, 7368816, 7434609, 7500402, 7566195, 7631988, 7697781, 7763574, 7829367, 7895160, 7960953, 8026746, 8092539, 8158332, 8224125, 8289918, 8355711, 8421504, 8487297, 8553090, 8618883, 8684676, 8750469, 8816262, 8882055, 8947848, 9013641, 9079434, 9145227, 9211020, 9276813, 9342606, 9408399, 9474192, 9539985, 9605778, 9671571, 9737364, 9803157, 9868950, 9934743, 10000536, 10066329, 10132122, 10197915, 10263708, 10329501, 10395294, 10461087, 10526880, 10592673, 10658466, 10724259, 10790052, 10855845, 10921638, 10987431, 11053224, 11119017, 11184810, 11250603, 11316396, 11382189, 11447982, 11513775, 11579568, 11645361, 11711154, 11776947, 11842740, 11908533, 11974326, 12040119, 12105912, 12171705, 12237498, 12303291, 12369084, 12434877, 12500670, 12566463, 12632256, 12698049, 12763842, 12829635, 12895428, 12961221, 13027014, 13092807, 13158600, 13224393, 13290186, 13355979, 13421772, 13487565, 13553358, 13619151, 13684944, 13750737, 13816530, 13882323, 13948116, 14013909, 14079702, 14145495, 14211288, 14277081, 14342874, 14408667, 14474460, 14540253, 14606046, 14671839, 14737632, 14803425, 14869218, 14935011, 15000804, 15066597, 15132390, 15198183, 15263976, 15329769, 15395562, 15461355, 15527148, 15592941, 15658734, 15724527, 15790320, 15856113, 15921906, 15987699, 16053492, 16119285, 16185078, 16250871, 16316664, 16382457, 16448250, 16514043, 16579836, 16645629, 16711422, 0] ("output array 2"), "8-bit pixmap"=w582) -> ("image data"=w577:T30)  [unwired: 9 in]
                                n258 = call <vilib>:"Write PNG File.vi"("image data"=w577, "path to PNG file"=w567) -> ()  [unwired: 8 in, 2 out]
                                n259 = Wait (ms)(milliseconds to wait=u32 300) -> ()  [unwired: 1 out]
                                }
                                }
                              }
                            }
                          }
                        }
                      }
                      n260 = Increment(x=w412) -> (x+1=→"Frame_X":i32)
                      "Total_Frame_Y" <- w413
                    }
                  }
                  frame #3 {
                    n261 = One Button Dialog(message="Scanning is finished!!!", button name ("OK")="OK") -> ()  [unwired: 1 out]
                  }
                }
              }
              event "X axis_R": Value Change {
                n262 = event-data() -> ()  [unwired: 1 in, 6 out]
                n263 = Unbundle(w594) -> ("Device X"=w592:refnum<k24>)  [unwired: 2 out]
                n264 = case shown="\"0.05mm\"" w586 {
                  tunnel: [0.01 0.1 0.5 1.0 1.5 0.05] -> w585
                  frame "0.01mm", Default {
                  }
                  frame "0.1mm" {
                  }
                  frame "0.5mm" {
                  }
                  frame "1mm" {
                  }
                  frame "1.5mm" {
                  }
                  frame "0.05mm" {
                  }
                }
                n265 = Subtract(x=12.0, y=w585) -> (x-y=w590:dbl)
                n266 = Greater?(x=w590, y=w589) -> (0:w588:bool)
                n267 = case shown="True" w588 {
                  tunnel: w592 -> [_ w607]
                  tunnel: w585 -> [_ w606]
                  frame False {
                  }
                  frame True {
                    w609 = 1 items=["Forward"=1, "Backward"=2] ("direction")
                    n268 = invoke class="KCubeDCServo" method="MoveRelative"(reference=w607, "direction"=w609, "stepSize"=w606, "waitTimeout"=0) -> ()  [unwired: 2 in, 6 out]
                  }
                }
                n269 = Wait (ms)(milliseconds to wait=u32 50) -> ()  [unwired: 1 out]
              }
              event "X axis_L": Value Change {
                n270 = event-data() -> ()  [unwired: 1 in, 6 out]
                n271 = Unbundle(w616) -> ("Device X"=w615:refnum<k24>)  [unwired: 2 out]
                n272 = case shown="\"0.05mm\"" w611 {
                  tunnel: [0.01 0.1 0.5 1.0 1.5 0.05] -> w610
                  frame "0.01mm", Default {
                  }
                  frame "0.1mm" {
                  }
                  frame "0.5mm" {
                  }
                  frame "1mm" {
                  }
                  frame "1.5mm" {
                  }
                  frame "0.05mm" {
                  }
                }
                n273 = Less?(x=w610, y=w614) -> (x < y?=w613:bool)
                n274 = case shown="True" w613 {
                  tunnel: w615 -> [_ w630]
                  tunnel: w610 -> [_ w629]
                  frame False {
                  }
                  frame True {
                    w632 = 2 items=["Forward"=1, "Backward"=2] ("direction")
                    n275 = invoke class="KCubeDCServo" method="MoveRelative"(reference=w630, "direction"=w632, "stepSize"=w629, "waitTimeout"=0) -> ()  [unwired: 2 in, 6 out]
                  }
                }
                n276 = Wait (ms)(milliseconds to wait=u32 50) -> ()  [unwired: 1 out]
              }
              event "Y axis_B": Value Change {
                n277 = event-data() -> ()  [unwired: 1 in, 6 out]
                n278 = Unbundle(w639) -> ("Device Y"=w638:refnum<k24>)  [unwired: 2 out]
                n279 = case shown="\"0.05mm\"" w634 {
                  tunnel: [0.01 0.1 0.5 1.0 1.5 0.05] -> w633
                  frame "0.01mm", Default {
                  }
                  frame "0.1mm" {
                  }
                  frame "0.5mm" {
                  }
                  frame "1mm" {
                  }
                  frame "1.5mm" {
                  }
                  frame "0.05mm" {
                  }
                }
                n280 = Subtract(x=12.0, y=w633) -> (x-y=w640:dbl)
                n281 = Greater?(x=w640, y=w636) -> (0:w637:bool)
                n282 = case shown="True" w637 {
                  tunnel: w638 -> [_ w655]
                  tunnel: w633 -> [_ w654]
                  frame False {
                  }
                  frame True {
                    w657 = 1 items=["Forward"=1, "Backward"=2] ("direction")
                    n283 = invoke class="KCubeDCServo" method="MoveRelative"(reference=w655, "direction"=w657, "stepSize"=w654, "waitTimeout"=0) -> ()  [unwired: 2 in, 6 out]
                  }
                }
                n284 = Wait (ms)(milliseconds to wait=u32 50) -> ()  [unwired: 1 out]
              }
              event "Y axis_F": Value Change {
                n285 = event-data() -> ()  [unwired: 1 in, 6 out]
                n286 = Unbundle(w663) -> ("Device Y"=w662:refnum<k24>)  [unwired: 2 out]
                n287 = case shown="\"0.05mm\"" w659 {
                  tunnel: [0.01 0.1 0.5 1.0 1.5 0.05] -> w658
                  frame "0.01mm", Default {
                  }
                  frame "0.1mm" {
                  }
                  frame "0.5mm" {
                  }
                  frame "1mm" {
                  }
                  frame "1.5mm" {
                  }
                  frame "0.05mm" {
                  }
                }
                n288 = Less?(x=w658, y=w661) -> (x < y?=w664:bool)
                n289 = case shown="True" w664 {
                  tunnel: w662 -> [_ w678]
                  tunnel: w658 -> [_ w677]
                  frame False {
                  }
                  frame True {
                    w680 = 2 items=["Forward"=1, "Backward"=2] ("direction")
                    n290 = invoke class="KCubeDCServo" method="MoveRelative"(reference=w678, "direction"=w680, "stepSize"=w677, "waitTimeout"=0) -> ()  [unwired: 2 in, 6 out]
                  }
                }
                n291 = Wait (ms)(milliseconds to wait=u32 50) -> ()  [unwired: 1 out]
              }
              event "Z axis_u": Value Change {
                n292 = event-data() -> ()  [unwired: 1 in, 6 out]
                n293 = Unbundle(w686) -> ("Device Z"=w685:refnum<k24>)  [unwired: 2 out]
                n294 = case shown="\"20step\"" w687 {
                  tunnel: [1 5 10 30 300 3000] -> w688
                  frame "1step", Default {
                  }
                  frame "2step" {
                  }
                  frame "5step" {
                  }
                  frame "10step" {
                  }
                  frame "15step" {
                  }
                  frame "20step" {
                  }
                }
                n295 = invoke class="KCubeDCServo" method="SetJogStepSize_DeviceUnit"(reference=w685, "stepSize"=w688) -> (reference out=w682:refnum<k24>)  [unwired: 2 in, 3 out]
                n296 = Less?(x=w683, y=11.5) -> (x < y?=w684:bool)
                n297 = case shown="True" w684 {
                  tunnel: w682 -> [_ w696]
                  frame False {
                  }
                  frame True {
                    w698 = 1 items=["Forward"=1, "Backward"=2] ("direction")
                    n298 = invoke class="KCubeDCServo" method="MoveJog"(reference=w696, "direction"=w698, "waitTimeout"=0) -> ()  [unwired: 2 in, 5 out]
                  }
                }
                n299 = Wait (ms)(milliseconds to wait=u32 50) -> ()  [unwired: 1 out]
              }
              event "Z axis_d": Value Change {
                n300 = event-data() -> ()  [unwired: 1 in, 6 out]
                n301 = Unbundle(w711) -> ("Device Z"=w712:refnum<k24>)  [unwired: 2 out]
                n302 = case shown="\"20step\"" w710 {
                  tunnel: [1 5 10 30 300 3000] -> w713
                  frame "1step", Default {
                  }
                  frame "2step" {
                  }
                  frame "5step" {
                  }
                  frame "10step" {
                  }
                  frame "15step" {
                  }
                  frame "20step" {
                  }
                }
                n303 = invoke class="KCubeDCServo" method="SetJogStepSize_DeviceUnit"(reference=w712, "stepSize"=w713) -> (reference out=w709:refnum<k24>)  [unwired: 2 in, 3 out]
                n304 = Less?(x=0.01 ("y"), y=w707) -> (x < y?=w708:bool)
                n305 = case shown="True" w708 {
                  tunnel: w709 -> [_ w720]
                  frame False {
                  }
                  frame True {
                    w722 = 2 items=["Forward"=1, "Backward"=2] ("direction")
                    n306 = invoke class="KCubeDCServo" method="MoveJog"(reference=w720, "direction"=w722, "waitTimeout"=0) -> ()  [unwired: 2 in, 5 out]
                  }
                }
                n307 = Wait (ms)(milliseconds to wait=u32 50) -> ()  [unwired: 1 out]
              }
              event "MoveTo": Value Change {
                n308 = event-data() -> ()  [unwired: 1 in, 6 out]
                n309 = Unbundle(w730) -> ("Device Z"=w729:refnum<k24>)  [unwired: 2 out]
                n310 = invoke class="KCubeDCServo" method="MoveTo"(reference=w729, "position"="Destination", "waitTimeout"=0) -> ()  [unwired: 2 in, 5 out]
                n311 = Wait (ms)(milliseconds to wait=u32 1000) -> ()  [unwired: 1 out]
              }
              event "Snap": Value Change {
                n312 = event-data() -> ()  [unwired: 1 in, 6 out]
                n313 = call "GetActImgMem.vi"("Camera Handle In"=w749) -> ("Image Memory Out"=w744:u8[])  [unwired: 7 in, 3 out]
                n314 = Unbundle(w742) -> ("Height"=w745:i32, "Width"=w746:i32)
                n315 = Reshape Array(w744, w745, w746) -> (w747:u8[][])
                n316 = call <vilib>:"Flatten Pixmap.vi"("colors"=u32[] [0, 65793, 131586, 197379, 263172, 328965, 394758, 460551, 526344, 592137, 657930, 723723, 789516, 855309, 921102, 986895, 1052688, 1118481, 1184274, 1250067, 1315860, 1381653, 1447446, 1513239, 1579032, 1644825, 1710618, 1776411, 1842204, 1907997, 1973790, 2039583, 2105376, 2171169, 2236962, 2302755, 2368548, 2434341, 2500134, 2565927, 2631720, 2697513, 2763306, 2829099, 2894892, 2960685, 3026478, 3092271, 3158064, 3223857, 3289650, 3355443, 3421236, 3487029, 3552822, 3618615, 3684408, 3750201, 3815994, 3881787, 3947580, 4013373, 4079166, 4144959, 4210752, 4276545, 4342338, 4408131, 4473924, 4539717, 4605510, 4671303, 4737096, 4802889, 4868682, 4934475, 5000268, 5066061, 5131854, 5197647, 5263440, 5329233, 5395026, 5460819, 5526612, 5592405, 5658198, 5723991, 5789784, 5855577, 5921370, 5987163, 6052956, 6118749, 6184542, 6250335, 6316128, 6381921, 6447714, 6513507, 6579300, 6645093, 6710886, 6776679, 6842472, 6908265, 6974058, 7039851, 7105644, 7171437, 7237230, 7303023, 7368816, 7434609, 7500402, 7566195, 7631988, 7697781, 7763574, 7829367, 7895160, 7960953, 8026746, 8092539, 8158332, 8224125, 8289918, 8355711, 8421504, 8487297, 8553090, 8618883, 8684676, 8750469, 8816262, 8882055, 8947848, 9013641, 9079434, 9145227, 9211020, 9276813, 9342606, 9408399, 9474192, 9539985, 9605778, 9671571, 9737364, 9803157, 9868950, 9934743, 10000536, 10066329, 10132122, 10197915, 10263708, 10329501, 10395294, 10461087, 10526880, 10592673, 10658466, 10724259, 10790052, 10855845, 10921638, 10987431, 11053224, 11119017, 11184810, 11250603, 11316396, 11382189, 11447982, 11513775, 11579568, 11645361, 11711154, 11776947, 11842740, 11908533, 11974326, 12040119, 12105912, 12171705, 12237498, 12303291, 12369084, 12434877, 12500670, 12566463, 12632256, 12698049, 12763842, 12829635, 12895428, 12961221, 13027014, 13092807, 13158600, 13224393, 13290186, 13355979, 13421772, 13487565, 13553358, 13619151, 13684944, 13750737, 13816530, 13882323, 13948116, 14013909, 14079702, 14145495, 14211288, 14277081, 14342874, 14408667, 14474460, 14540253, 14606046, 14671839, 14737632, 14803425, 14869218, 14935011, 15000804, 15066597, 15132390, 15198183, 15263976, 15329769, 15395562, 15461355, 15527148, 15592941, 15658734, 15724527, 15790320, 15856113, 15921906, 15987699, 16053492, 16119285, 16185078, 16250871, 16316664, 16382457, 16448250, 16514043, 16579836, 16645629, 16711422, 0] ("output array 2"), "8-bit pixmap"=w747) -> ("image data"=w741:T30)  [unwired: 9 in]
                n317 = call <vilib>:"Write PNG File.vi"("image data"=w741) -> ()  [unwired: 9 in, 2 out]
              }
              event "Scan Mode": Value Change {
                n318 = event-data() -> ()  [unwired: 1 in, 6 out]
                n319 = local read "ZOffset"() -> (w761:dbl)
                n320 = call "h_0.35_2"() -> ("Signal"=w763:dynamicdata)  [unwired: 9 in, 2 out]
                n321 = call <vilib>:"DAQmx Start Task.vi"("task/channels in"=w757, "error in"=w755) -> ("task out"=w756:refnum<k21>, "error out"=w754:errorcluster)  [unwired: 12 in]
                n322 = call "ao2"("Offset"=w761) -> ("DC"=w762:dynamicdata)  [unwired: 13 in, 1 out]
                n323 = call "ao4"() -> ("Signal"=w764:dynamicdata)  [unwired: 9 in, 2 out]
                n324 = Build Array(w764, w763, w762) -> (w760:dynamicdata[])
                n325 = call "Galvo_Reset.vi"("error in"=w754, "auto start"=FALSE, "Signal array"=w760, "task/channels in"=w756) -> ("error out"=w759:errorcluster, "task out"=w765:refnum<k21>)  [unwired: 6 in]
              }
              event "Galvo DC": Value Change {
                n326 = event-data() -> ()  [unwired: 1 in, 6 out]
                n327 = local read "ZOffset"() -> (w784:dbl)
                n328 = call "ao7"("Offset"="YOffset") -> ("DC"=w781:dynamicdata)  [unwired: 13 in, 1 out]
                n329 = call "ao6"("Offset"="XOffset") -> ("DC"=w782:dynamicdata)  [unwired: 13 in, 1 out]
                n330 = call "ao5"("Offset"=w784) -> ("DC"=w785:dynamicdata)  [unwired: 13 in, 1 out]
                n331 = call <vilib>:"DAQmx Start Task.vi"("task/channels in"=w778, "error in"=w776) -> ("task out"=w777:refnum<k21>, "error out"=w775:errorcluster)  [unwired: 12 in]
                n332 = Build Array(w782, w781, w785) -> (w783:dynamicdata[])
                n333 = call "Galvo_Reset.vi"("error in"=w775, "auto start"=TRUE, "Signal array"=w783, "task/channels in"=w777) -> ("error out"=w772:errorcluster, "task out"=w773:refnum<k21>)  [unwired: 6 in]
                n334 = call <vilib>:"DAQmx Stop Task.vi"("task/channels in"=w773, "error in"=w772) -> ("task out"=w771:refnum<k21>, "error out"=w770:errorcluster)  [unwired: 12 in]
              }
              event "Live video": Mouse Down {
                # "When the mouse is inside the video area, after the mouse is down and hold, the coordinate of the ROI upper left corner is stored."
                n335 = event-data() -> ("Coords"=w794:T20)  [unwired: 1 in, 7 out]
              }
              event "Live video": Mouse Up {
                # "When the mouse is inside the video area, after the mouse is up, the edge of the ROI is calculated."
                n336 = event-data() -> ("Coords"=w803:T20)  [unwired: 1 in, 7 out]
                n337 = property on="Live video" class="Pict"() -> ("Position"=w801:T31)  [unwired: 2 in, 2 out]
                n338 = Unbundle By Name "Start"(w802) -> ("Horizontal"=w823:i32, "Vertical"=w820:i32)
                n339 = Unbundle By Name(w803) -> ("Horizontal"=w817:i32, "Vertical"=w814:i32)
                n340 = Unbundle By Name(w801) -> ("Left"=w825:i32, "Top"=w824:i32)
                n341 = Subtract(x=w823, y=3) -> (x-y=w821:i32)
                n342 = Subtract(x=w820, y=3) -> (x-y=w819:i32)
                n343 = Subtract(x=w817, y=3) -> (x-y=w815:i32)
                n344 = Subtract(x=w814, y=3) -> (x-y=w812:i32)
                n345 = Subtract(x=w821, y=w825) -> (x-y=w811:i32)
                n346 = Subtract(x=w819, y=w824) -> (x-y=w810:i32)
                n347 = Subtract(x=w815, y=w825) -> (x-y=w797:i32)
                n348 = Subtract(x=w812, y=w824) -> (x-y=w796:i32)
                n349 = Divide(x=w811, y=w804) -> (x/y=w809:dbl)
                n350 = Divide(x=w810, y=w804) -> (x/y=w808:dbl)
                n351 = Divide(x=w797, y=w804) -> (x/y=w807:dbl)
                n352 = Divide(x=w796, y=w804) -> (x/y=w806:dbl)
                n353 = Bundle By Name(cluster=T19 {"left"=0, "top"=0, "right"=0, "bottom"=0} ("rect"), "left"=w809, "top"=w808, "right"=w807, "bottom"=w806) -> (w805:T19)
              }
              event "Quit": Value Change {
                # "Add recover initial position\nZ: max\nX: middle\nY: middle\nand also need to attch a limit"
                # "When user clicks the STOP button, program will jump to \"Shut down\" state"
                n354 = event-data() -> ()  [unwired: 1 in, 6 out]
              }
              event "Focus": Value Change {
                # "When clicking the Focus button, following steps will be executed: \n1. move the stage to 4 different Z positions and take an image at each position;\n2. crop the image to get 4 ROIs and use them to find the focal plane;\n3. move the stage to the focal plane."
                n355 = event-data() -> ()  [unwired: 1 in, 6 out]
                n356 = Divide(x="Jog size (um)", y=1000.0) -> (x/y=w836:dbl)
                n357 = Divide(x=w836, y=2.0) -> (x/y=w838:dbl)
                n358 = call "StageReadPos.vi"("error in (no error)"=w879, "Stage Select"=StageSelect."Z axis", "Device In"=w850) -> ("error out"=w877:errorcluster, "CurrentPosition"=w843:dbl)  [unwired: 7 in]
                n359 = Unbundle By Name(w872) -> ("Device Z"=w869:refnum<k24>)
                n360 = Add(x=w843, y=w836) -> (x+y=w841:dbl)
                n361 = Subtract(x=w843, y=w836) -> (x-y=w873:dbl)
                n362 = invoke class="KCubeDCServo" method="GetVelocityParams"(reference=w869) -> ("GetVelocityParams"=w868:refnum<k24>)  [unwired: 2 in, 2 out]
                n363 = Subtract(x=w843, y=w838) -> (x-y=w844:dbl)
                n364 = Subtract(x=w841, y=w838) -> (x-y=w842:dbl)
                n365 = Add(x=w842, y=w836) -> (x+y=w839:dbl)
                n366 = Subtract(x=w873, y=w838) -> (x-y=w837:dbl)
                n367 = Subtract(x=w839, y=w838) -> (x-y=w840:dbl)
                n368 = Build Array(w837, w844, w842, w840) -> (w870:dbl[])
                n369 = property class="VelocityParameters"(reference=w868) -> (reference out=w866:refnum<k24>, error out=w867:errorcluster, "Acceleration"=w865:dbl)  [unwired: 1 in]
                n370 = property class="VelocityParameters"(reference=w866, error in=w867) -> ("MaxVelocity"=w864:dbl)  [unwired: 2 out]
                n371 = for {
                  tunnel: w870 -> [w908] mode=indexing
                  tunnel: w877 -> [w911]
                  tunnel: w850 -> [w910]
                  tunnel: [w901] -> w871
                  tunnel: w876 -> [w904]
                  tunnel: w875 -> [w903]
                  tunnel: [w883] -> w859 mode=indexing
                  tunnel: w874 -> [w899]
                  tunnel: w836 -> [w897]
                  tunnel: w865 -> [w888]
                  tunnel: w864 -> [w887]
                  w891 = 0.9 ("y")
                  n372 = call "StageToPos.vi"("error in (no error)"=w911, "Move to pos"=w908, "Stage Select"=StageSelect."Z axis", "Device In"=w910) -> ("error out"=w896:errorcluster)  [unwired: 7 in]
                  n373 = call "MovingTime.vi"("error in"=w896, "Acc (mm/s^2)"=w888, "MaxV (mm/s)"=w887, "Distance (mm)"=w897) -> ("error out"=w895:errorcluster, "time (s)"=w894:dbl)  [unwired: 6 in]
                  n374 = Multiply(x=w894, y=2.0) -> (x*y=w890:dbl)
                  n375 = Greater?(x=w890, y=w891) -> (0:w892:bool)
                  n376 = Select(t=w890, s=w892, f=w891) -> (s? t:f=w889:dbl)
                  "Delay (s)" <- w889
                  n377 = call "Time Delay"("error in (no error)"=w895, "Delay Time (s)"=w889) -> ("error out"=w898:errorcluster)  [unwired: 9 in]
                  n378 = call "GetActImgMem.vi"("error in"=w898, "Camera Handle In"=w904) -> ("error out"=w902:errorcluster, "Image Memory Out"=w905:u8[])  [unwired: 6 in, 2 out]
                  n379 = Unbundle(w903) -> ("Height"=w906:i32, "Width"=w907:i32)
                  n380 = Reshape Array(w905, w906, w907) -> (w882:u8[][])
                  n381 = call <vilib>:"Flatten Pixmap.vi"("colors"=u32[] [0, 65793, 131586, 197379, 263172, 328965, 394758, 460551, 526344, 592137, 657930, 723723, 789516, 855309, 921102, 986895, 1052688, 1118481, 1184274, 1250067, 1315860, 1381653, 1447446, 1513239, 1579032, 1644825, 1710618, 1776411, 1842204, 1907997, 1973790, 2039583, 2105376, 2171169, 2236962, 2302755, 2368548, 2434341, 2500134, 2565927, 2631720, 2697513, 2763306, 2829099, 2894892, 2960685, 3026478, 3092271, 3158064, 3223857, 3289650, 3355443, 3421236, 3487029, 3552822, 3618615, 3684408, 3750201, 3815994, 3881787, 3947580, 4013373, 4079166, 4144959, 4210752, 4276545, 4342338, 4408131, 4473924, 4539717, 4605510, 4671303, 4737096, 4802889, 4868682, 4934475, 5000268, 5066061, 5131854, 5197647, 5263440, 5329233, 5395026, 5460819, 5526612, 5592405, 5658198, 5723991, 5789784, 5855577, 5921370, 5987163, 6052956, 6118749, 6184542, 6250335, 6316128, 6381921, 6447714, 6513507, 6579300, 6645093, 6710886, 6776679, 6842472, 6908265, 6974058, 7039851, 7105644, 7171437, 7237230, 7303023, 7368816, 7434609, 7500402, 7566195, 7631988, 7697781, 7763574, 7829367, 7895160, 7960953, 8026746, 8092539, 8158332, 8224125, 8289918, 8355711, 8421504, 8487297, 8553090, 8618883, 8684676, 8750469, 8816262, 8882055, 8947848, 9013641, 9079434, 9145227, 9211020, 9276813, 9342606, 9408399, 9474192, 9539985, 9605778, 9671571, 9737364, 9803157, 9868950, 9934743, 10000536, 10066329, 10132122, 10197915, 10263708, 10329501, 10395294, 10461087, 10526880, 10592673, 10658466, 10724259, 10790052, 10855845, 10921638, 10987431, 11053224, 11119017, 11184810, 11250603, 11316396, 11382189, 11447982, 11513775, 11579568, 11645361, 11711154, 11776947, 11842740, 11908533, 11974326, 12040119, 12105912, 12171705, 12237498, 12303291, 12369084, 12434877, 12500670, 12566463, 12632256, 12698049, 12763842, 12829635, 12895428, 12961221, 13027014, 13092807, 13158600, 13224393, 13290186, 13355979, 13421772, 13487565, 13553358, 13619151, 13684944, 13750737, 13816530, 13882323, 13948116, 14013909, 14079702, 14145495, 14211288, 14277081, 14342874, 14408667, 14474460, 14540253, 14606046, 14671839, 14737632, 14803425, 14869218, 14935011, 15000804, 15066597, 15132390, 15198183, 15263976, 15329769, 15395562, 15461355, 15527148, 15592941, 15658734, 15724527, 15790320, 15856113, 15921906, 15987699, 16053492, 16119285, 16185078, 16250871, 16316664, 16382457, 16448250, 16514043, 16579836, 16645629, 16711422, 0] ("output array 2"), "8-bit pixmap"=w882) -> ("image data"=w886:T30)  [unwired: 9 in]
                  n382 = call <vilib>:"Draw Flattened Pixmap.vi"("image data"=w886) -> ("new picture"=w884:picture)  [unwired: 8 in]
                  n383 = local write "Live video"(w884) -> ()
                  n384 = call "ROI_crop.vi"("error constant"=w902, "roiEdge"=w899, "InputImage"=w882) -> ("error constant 2"=w901:errorcluster, "ROI"=w900:dbl[][])  [unwired: 7 in]
                  n385 = To Unsigned Byte Integer(number=w900) -> (unsigned 8bit integer=w883:u8[][])
                }
                n386 = Index Array(array=w859, index (dim 0)=0 ("index (page)")) -> (element=w857:u8[][])  [unwired: 2 in]
                n387 = Index Array(array=w859, index (dim 0)=1 ("index (page)")) -> (element=w856:u8[][])  [unwired: 2 in]
                n388 = Index Array(array=w859, index (dim 0)=2 ("index (page)")) -> (element=w855:u8[][])  [unwired: 2 in]
                n389 = Index Array(array=w859, index (dim 0)=3 ("index (page)")) -> (element=w854:u8[][])  [unwired: 2 in]
                n390 = Bundle By Name(cluster=T27 {"Image2"=[], "Image3"=[], "Image4"=[], "Image1"=[]} ("Imput images"), "Image1"=w857, "Image2"=w856, "Image3"=w855, "Image4"=w854) -> (w853:T27)
                n391 = call "Find_Focus.vi"("error in (no error)"=w871, "Input_Z"=w870, "Imput images"=w853) -> ("error out"=w852:errorcluster, "BestPosition"=w848:dbl)  [unwired: 7 in]
                "Focal plane (mm)" <- w848
                n392 = call "StageToPos.vi"("error in (no error)"=w852, "Move to pos"=w848, "Stage Select"=StageSelect."Z axis", "Device In"=w850) -> ("error out"=w851:errorcluster)  [unwired: 7 in]
              }
              event "Aim": Value Change {
                # "First, you need to draw an ROI, and then when you click the Aim button, the center of the\nview will move to the center of the selected ROI."
                n393 = event-data() -> ()  [unwired: 1 in, 6 out]
                n394 = Unbundle By Name(w948) -> ("left"=w946:i16, "right"=w947:i16, "top"=w941:i16, "bottom"=w940:i16)
                n395 = Unbundle By Name(w914) -> ("Laser X"=w913:dbl, "Laser Y"=w912:dbl)
                n396 = Add(x=w946, y=w947) -> (x+y=w945:i16)
                n397 = Add(x=w941, y=w940) -> (x+y=w942:i16)
                n398 = Divide(x=w945, y=i16 2) -> (x/y=w939:dbl)
                n399 = Divide(x=w942, y=i16 2) -> (x/y=w938:dbl)
                n400 = Subtract(x=w939, y=w913) -> (x-y=w928:dbl)
                n401 = Subtract(x=w938, y=w912) -> (x-y=w933:dbl)
                n402 = Divide(x="Pixel Size Y (um)", y=1000.0) -> (x/y=w929:dbl)
                n403 = Divide(x="Pixel Size X (um)", y=1000.0) -> (x/y=w927:dbl)
                n404 = Multiply(x=w927, y=w928) -> (x*y=w934:dbl)
                n405 = Multiply(x=w933, y=w929) -> (x*y=w932:dbl)
                n406 = call "StageReadPos.vi"("error in (no error)"=w949, "Stage Select"=StageSelect."X axis", "Device In"=w937) -> ("error out"=w926:errorcluster, "CurrentPosition"=w923:dbl)  [unwired: 7 in]
                n407 = call "StageReadPos.vi"("error in (no error)"=w949, "Stage Select"=StageSelect."Y axis", "Device In"=w937) -> ("error out"=w919:errorcluster, "CurrentPosition"=w918:dbl)  [unwired: 7 in]
                n408 = Add(x=w932, y=w918) -> (x+y=w917:dbl)
                n409 = Add(x=w934, y=w923) -> (x+y=w922:dbl)
                n410 = call "StageToPos.vi"("error in (no error)"=w926, "Move to pos"=w922, "Stage Select"=StageSelect."X axis", "Device In"=w937) -> ("error out"=w916:errorcluster)  [unwired: 7 in]
                n411 = call "StageToPos.vi"("error in (no error)"=w919, "Move to pos"=w917, "Stage Select"=StageSelect."Y axis", "Device In"=w937) -> ("error out"=w915:errorcluster)  [unwired: 7 in]
                n412 = Merge Errors(w916, w915) -> (w950:errorcluster)
              }
              event "LaserSpot": Value Change {
                # "First, you need to draw an ROI, and then when you click the Here's Laser button, the center of the\nROI will be stored for Aim use."
                n413 = event-data() -> ()  [unwired: 1 in, 6 out]
                n414 = Unbundle By Name(w959) -> ("left"=w966:i16, "right"=w967:i16, "top"=w961:i16, "bottom"=w960:i16)
                n415 = Add(x=w966, y=w967) -> (x+y=w965:i16)
                n416 = Add(x=w961, y=w960) -> (x+y=w962:i16)
                n417 = Divide(x=w965, y=i16 2) -> (x/y=w955:dbl)
                n418 = Divide(x=w962, y=i16 2) -> (x/y=w954:dbl)
                n419 = Bundle By Name(cluster=T18 {"Laser X"=0.0, "Laser Y"=0.0} ("LaserSpot"), "Laser X"=w955, "Laser Y"=w954) -> (w957:T18)
                n420 = local write "Spot X"(w955) -> ()
                n421 = local write "Spot Y"(w954) -> ()
                "Boolean" <- TRUE ("Boolean")
              }
              event "Left": Value Change {
                n422 = event-data() -> ()  [unwired: 1 in, 6 out]
                n423 = Unbundle By Name(w975) -> ("Laser X"=w973:dbl, "Laser Y"=w974:dbl)
                n424 = Decrement(x=w973) -> (x-1=w972:dbl)
                n425 = Bundle By Name(cluster=T18 {"Laser X"=0.0, "Laser Y"=0.0} ("LaserSpot"), "Laser X"=w972, "Laser Y"=w974) -> (w976:T18)
                n426 = local write "Spot X"(w972) -> ()
              }
              event "Right": Value Change {
                n427 = event-data() -> ()  [unwired: 1 in, 6 out]
                n428 = Unbundle By Name(w986) -> ("Laser X"=w984:dbl, "Laser Y"=w987:dbl)
                n429 = Increment(x=w984) -> (x+1=w983:dbl)
                n430 = Bundle By Name(cluster=T18 {"Laser X"=0.0, "Laser Y"=0.0} ("LaserSpot"), "Laser X"=w983, "Laser Y"=w987) -> (w985:T18)
                n431 = local write "Spot X"(w983) -> ()
              }
              event "Up": Value Change {
                n432 = event-data() -> ()  [unwired: 1 in, 6 out]
                n433 = Unbundle By Name(w998) -> ("Laser X"=w996:dbl, "Laser Y"=w995:dbl)
                n434 = Decrement(x=w995) -> (x-1=w994:dbl)
                n435 = Bundle By Name(cluster=T18 {"Laser X"=0.0, "Laser Y"=0.0} ("LaserSpot"), "Laser X"=w996, "Laser Y"=w994) -> (w997:T18)
                n436 = local write "Spot Y"(w994) -> ()
              }
              event "Down": Value Change {
                n437 = event-data() -> ()  [unwired: 1 in, 6 out]
                n438 = Unbundle By Name(w1009) -> ("Laser X"=w1007:dbl, "Laser Y"=w1006:dbl)
                n439 = Increment(x=w1006) -> (x+1=w1005:dbl)
                n440 = Bundle By Name(cluster=T18 {"Laser X"=0.0, "Laser Y"=0.0} ("LaserSpot"), "Laser X"=w1007, "Laser Y"=w1005) -> (w1008:T18)
                n441 = local write "Spot Y"(w1005) -> ()
              }
              event "Galvo Scan": Value Change {
                w1017 = T24."Disabled and Grayed Out" ("Disabled")
                n442 = event-data() -> ()  [unwired: 1 in, 6 out]
                n443 = flat-sequence {
                  tunnel: w1024 -> [w1028]
                  tunnel: [w1028] -> w1016
                  tunnel: w1025 -> [w1033]
                  tunnel: [w1031] -> w1020
                  tunnel: [w1030] -> w1019
                  tunnel: [TRUE] -> w1018
                  tunnel: w1016 -> [w1032]
                  frame #0 {
                    n444 = Wait Until Next ms Multiple(millisecond multiple="Delay/ms") -> ()  [unwired: 1 out]
                  }
                  frame #1 {
                    n445 = call <vilib>:"DAQmx Start Task.vi"("task/channels in"=w1033, "error in"=w1032) -> ("task out"=w1031:refnum<k21>, "error out"=w1030:errorcluster)  [unwired: 12 in]
                  }
                }
                n446 = property on="Galvo Scan" class="Bool"("DisabledEnum"=w1017) -> ()  [unwired: 2 in, 2 out]
                n447 = property on="Galvo DC" class="Bool"("DisabledEnum"=w1017) -> ()  [unwired: 2 in, 2 out]
                n448 = property on="Scan Mode" class="Bool"("DisabledEnum"=w1017) -> ()  [unwired: 2 in, 2 out]
                "Galvo" <- w1018
              }
              event "Galvo Stop": Value Change {
                w1034 = T24."Enabled" ("Disabled")
                n449 = event-data() -> ()  [unwired: 1 in, 6 out]
                n450 = call <vilib>:"DAQmx Stop Task.vi"("task/channels in"=w1037, "error in"=w1035) -> ("error out"=w1036:errorcluster)  [unwired: 12 in, 1 out]
                n451 = property on="Scan Mode" class="Bool"("DisabledEnum"=w1034) -> ()  [unwired: 2 in, 2 out]
                n452 = property on="Galvo Scan" class="Bool"("DisabledEnum"=w1034) -> ()  [unwired: 2 in, 2 out]
                n453 = property on="Galvo DC" class="Bool"("DisabledEnum"=w1034) -> ()  [unwired: 2 in, 2 out]
              }
            }
          }
        }
      }
      n454 = call <vilib>:"Simple Error Handler.vi"("error in (no error)"=w10) -> ()  [unwired: 4 in, 5 out]
    }
  }
  n455 = while {
    stop <- w1042 stop-if-true
    n456 = local read "Initialization finished"() -> (w1043:bool)
    n457 = case shown="True" w1043 {
      tunnel: [FALSE ("ShutDown") w1045] -> w1042
      frame False {
      }
      frame True {
        n458 = while {
          shift-right: [w1051] -> _
          shift-left: enum16{"Initialize", "Live", "Exit"}."Initialize" -> [w1052]
          shift-right: [w1049] -> _
          shift-left: errorcluster {"status"=FALSE, "code"=0, "source"=""} ("error in") -> [w1050]
          tunnel: [w1048] -> w1045
          stop <- w1048 stop-if-true
          n459 = case shown="\"Live\"" w1052 {
            tunnel: [enum16{"Initialize", "Live", "Exit"}."Live" w1094 enum16{"Initialize", "Live", "Exit"}."Exit"] -> w1051
            tunnel: w1050 -> [w1057 w1093 w1180]
            tunnel: [w1054 w1092 w1179] -> w1049
            tunnel: [FALSE ("ShutDown") FALSE ("ShutDown") w1171] -> w1048
            frame "Initialize", Default {
              n460 = flat-sequence {
                tunnel: [w1066] -> w1058
                tunnel: w1057 -> [w1066]
                tunnel: w1058 -> [w1080]
                tunnel: [w1079] -> w1056
                tunnel: w1056 -> [w1088]
                tunnel: [w1087] -> w1055
                tunnel: w1055 -> [w1089]
                tunnel: [w1089] -> w1054
                frame #0 {
                  n461 = local write "ShutDown"(cluster{"CoolOff":bool, "ShutDown":bool} {"CoolOff"=FALSE, "ShutDown"=FALSE} ("ShutDown")) -> ()
                  n462 = local write "SetStatus"(FALSE ("SetStatus")) -> ()
                  n463 = local write "GetStatus"(T16 {"GetDetector"=FALSE, "GetHardVer"=FALSE, "GetNVS"=FALSE, "GetVS"=FALSE, "GetSotfVer"=FALSE, "GetNHS"=FALSE, "GetHS"=FALSE} ("GetStatus")) -> ()
                  n464 = local write "SaveStatus"(FALSE ("Save")) -> ()
                  n465 = local write "CoolerON"(T15 {"SetTemp"=FALSE, "CoolerOn"=FALSE, "Stablized"=FALSE} ("CoolerON")) -> ()
                  n466 = local write "DevInit"(FALSE ("DevInit")) -> ()
                }
                frame #1 {
                  n467 = local read "TargetTemp"() -> (w1075:i32)
                  n468 = control-ref of="CurrentTemp"() -> (w1077:refnum<vi>)
                  n469 = control-ref of="GetStatus"() -> (w1078:refnum<vi>)
                  n470 = control-ref of="CoolerON"() -> (w1076:refnum<vi>)
                  n471 = call "AndorInit.vi"("TargetTemp"=w1075, "error in"=w1080, "CoolerONRef"=w1076, "GetStatusRef"=w1078, "CurrentTempRef"=w1077) -> ("GetStatus"=w1067:T16, "CurrentTemp"=w1074:i32, "CoolerON"=w1073:T15, "DevInit"=w1070:bool, "DevSize"=w1069:cluster{"xpixels":i32, "ypixels":i32}, "HardWVersion"=w1068:T12, "SoftWVersion"=w1071:T13, "Speeds"=w1072:T14, "error out"=w1079:errorcluster)  [unwired: 6 in]
                  n472 = local write "CurrentTemp"(w1074) -> ()
                  n473 = local write "SoftWVersion"(w1071) -> ()
                  n474 = local write "Speeds"(w1072) -> ()
                  n475 = local write "HardWVersion"(w1068) -> ()
                  n476 = local write "DevSize"(w1069) -> ()
                  n477 = local write "DevInit"(w1070) -> ()
                  n478 = local write "GetStatus"(w1067) -> ()
                  n479 = local write "CoolerON"(w1073) -> ()
                }
                frame #2 {
                  n480 = local read "MultiTrack"() -> (w1084:cluster{"StartRow":i32, "EndRow":i32})
                  n481 = local read "AcqSet"() -> (w1086:T9)
                  n482 = local read "Mode"() -> (w1085:T8)
                  n483 = call "AndorSet.vi"("error in"=w1088, "MultiTrack"=w1084, "AcqSet"=w1086, "Mode"=w1085) -> ("error out"=w1087:errorcluster, "SetStatus"=w1081:bool, "SetOut"=w1082:T11, "Timing"=w1083:T10)  [unwired: 4 in]
                  n484 = local write "SetOut"(w1082) -> ()
                  n485 = local write "Timing"(w1083) -> ()
                  n486 = local write "SetStatus"(w1081) -> ()
                }
                frame #3 {
                }
              }
            }
            frame "Live" {
              n487 = event shown="[3] \"Galvo Scan\": Value Change" {
                selector: _ -> [_ _ _ _ _]
                dyn-events: _ -> [_ _ _ _ _]
                timeout: 0 -> [_ _ _ _ _]
                tunnel: [enum16{"Initialize", "Live", "Exit"}."Live" enum16{"Initialize", "Live", "Exit"}."Live" enum16{"Initialize", "Live", "Exit"}."Live" enum16{"Initialize", "Live", "Exit"}."Live" enum16{"Initialize", "Live", "Exit"}."Exit"] -> w1094
                tunnel: w1093 -> [w1096 w1107 w1111 w1138 w1169]
                tunnel: [w1095 w1106 w1109 w1135 w1169] -> w1092
                event Timeout {
                  n488 = event-data() -> ()  [unwired: 1 in, 3 out]
                  n489 = call <userlib>:"GetTemperature.vi"("error in (no error)"=w1096) -> ("error out"=w1095:errorcluster, "temperature"=w1098:i32)  [unwired: 3 in, 2 out]
                  n490 = local write "CurrentTemp"(w1098) -> ()
                  n491 = Wait Until Next ms Multiple(millisecond multiple=u32 500) -> ()  [unwired: 1 out]
                }
                event "Set": Value Change {
                  n492 = event-data() -> ()  [unwired: 1 in, 6 out]
                  n493 = local read "AcqSet"() -> (w1104:T9)
                  n494 = local read "MultiTrack"() -> (w1103:cluster{"StartRow":i32, "EndRow":i32})
                  n495 = local read "Mode"() -> (w1105:T8)
                  n496 = call "AndorSet.vi"("error in"=w1107, "MultiTrack"=w1103, "AcqSet"=w1104, "Mode"=w1105) -> ("error out"=w1106:errorcluster, "SetStatus"=w1101:bool, "SetOut"=w1100:T11, "Timing"=w1102:T10)  [unwired: 4 in]
                  n497 = local write "Timing"(w1102) -> ()
                  n498 = local write "SetStatus"(w1101) -> ()
                  n499 = local write "SetOut"(w1100) -> ()
                }
                event "AndorSnap": Value Change {
                  n500 = event-data() -> ()  [unwired: 1 in, 6 out]
                  n501 = flat-sequence {
                    tunnel: w1111 -> [w1117]
                    tunnel: [w1114] -> w1112
                    tunnel: w1112 -> [w1129]
                    tunnel: [TRUE ("SaveStatus")] -> w1110
                    tunnel: [w1126] -> w1109
                    frame #0 {
                      n502 = case shown="No Error" w1117 {
                        tunnel: w1117 -> [w1120 w1125]
                        tunnel: [w1118 FALSE ("SaveStatus")] -> w1116
                        tunnel: [w1119 w1125] -> w1114
                        frame No Error {
                          n503 = local read "AcqSet"() -> (w1122:T9)
                          n504 = Unbundle By Name(w1122) -> ("KineticNum"=w1121:i32)
                          n505 = call "AndorSaveasSif.vi"("error in"=w1120, "KinNumber"=w1121, "FilePath"="FilePath") -> ("error out"=w1119:errorcluster, "SaveStatus"=w1118:bool)  [unwired: 7 in]
                        }
                        frame Error {
                        }
                      }
                      n506 = Not(x=w1116) -> (.not. x?=→"SaveStatus":bool)
                    }
                    frame #1 {
                      n507 = call <userlib>:"StartAcquisition.vi"("error in (no error)"=w1129) -> ("error out"=w1128:errorcluster)  [unwired: 1 in, 1 out]
                      n508 = while {
                        tunnel: w1128 -> [w1134]
                        tunnel: [w1131] -> w1126
                        stop <- w1130 continue-if-true
                        n509 = call <userlib>:"GetStatus.vi"("error in (no error)"=w1134) -> ("error out"=w1131:errorcluster, "status"=w1133:T32)  [unwired: 2 in, 1 out]
                        n510 = Equal?(x=w1133, y=Error_Code_Enum_typedef."DRV_ACQUIRING") -> (x = y?=w1130:bool)
                      }
                    }
                  }
                  n511 = local write "SaveStatus"(w1110) -> ()
                }
                event "Galvo Scan": Value Change {
                  n512 = event-data() -> ()  [unwired: 1 in, 6 out]
                  n513 = flat-sequence {
                    tunnel: w1138 -> [w1144]
                    tunnel: [w1143] -> w1137
                    tunnel: [w1156] -> w1139
                    tunnel: w1137 -> [w1154]
                    tunnel: [TRUE ("SaveStatus")] -> w1136
                    tunnel: w1139 -> [w1166]
                    tunnel: w1136 -> [w1167]
                    tunnel: [w1166] -> w1135
                    frame #0 {
                      n514 = case shown="Error" w1144 {
                        tunnel: [w1147 FALSE ("SaveStatus")] -> w1142
                        tunnel: [w1148 w1151] -> w1143
                        tunnel: w1144 -> [w1145 w1151]
                        frame No Error {
                          n515 = local read "FilePath"() -> (w1146:string)
                          n516 = local read "AcqSet"() -> (w1150:T9)
                          n517 = Unbundle By Name(w1150) -> ("KineticNum"=w1149:i32)
                          n518 = call "AndorSaveasSif.vi"("error in"=w1145, "KinNumber"=w1149, "FilePath"=w1146) -> ("error out"=w1148:errorcluster, "SaveStatus"=w1147:bool)  [unwired: 7 in]
                        }
                        frame Error {
                        }
                      }
                      n519 = Not(x=w1142) -> (.not. x?=w1141:bool)
                      n520 = local write "SaveStatus"(w1141) -> ()
                      n521 = local write "Andor"(w1141) -> ()
                    }
                    frame #1 {
                      n522 = flat-sequence {
                        tunnel: [w1160] -> w1157
                        tunnel: [TRUE] -> w1155
                        tunnel: w1154 -> [w1158]
                        frame #0 {
                          n523 = call <userlib>:"StartAcquisition.vi"("error in (no error)"=w1158) -> ("error out"=w1160:errorcluster)  [unwired: 1 in, 1 out]
                        }
                      }
                      n524 = local write "Andor"(w1155) -> ()
                      n525 = while {
                        tunnel: w1157 -> [w1165]
                        tunnel: [w1162] -> w1156
                        stop <- w1161 continue-if-true
                        n526 = call <userlib>:"GetStatus.vi"("error in (no error)"=w1165) -> ("error out"=w1162:errorcluster, "status"=w1164:T32)  [unwired: 2 in, 1 out]
                        n527 = Equal?(x=w1164, y=Error_Code_Enum_typedef."DRV_ACQUIRING") -> (x = y?=w1161:bool)
                        "Andor" <- w1161
                      }
                    }
                    frame #2 {
                      n528 = local write "SaveStatus"(w1167) -> ()
                      n529 = local write "Galvo"(FALSE ("Galvo")) -> ()
                    }
                  }
                }
                event "Exit": Value Change {
                  n530 = event-data() -> ()  [unwired: 1 in, 6 out]
                }
              }
            }
            frame "Exit" {
              n531 = local read "CoolerON"() -> (w1178:T15)
              n532 = Unbundle By Name(w1178) -> ("SetTemp"=w1177:bool, "CoolerOn"=w1176:bool)
              n533 = control-ref of="CurrentTemp"() -> (w1175:refnum<vi>)
              n534 = control-ref of="ShutDown"() -> (w1173:refnum<vi>)
              n535 = call "AndorShutdown.vi"("ShutDownRef"=w1173, "CurrentTempRef"=w1175, "error in"=w1180, "CoolerON"=w1176, "SetTemp"=w1177) -> ("error out"=w1179:errorcluster, "ShutDown"=w1172:cluster{"CoolOff":bool, "ShutDown":bool}, "CurrentTemp"=w1174:i32)  [unwired: 4 in]
              "ShutDown" <- w1172
              n536 = local write "CurrentTemp"(w1174) -> ()
              n537 = Unbundle By Name(w1172) -> ("ShutDown"=w1171:bool)  [unwired: 1 out]
            }
          }
        }
      }
    }
  }
